vi "Rejestrator2_stare.vi"() -> ()   [LabVIEW 2014]
uses:
  C:/Users/user/Documents/Rudpol2/Kontrolki/GUI/AI_parametry.ctl
  C:/Users/user/Documents/Rudpol2/Kontrolki/GUI/AI_wartosc.ctl
  C:/Users/user/Documents/Rudpol2/Kontrolki/KartaDAQ/CONF AI HW config.ctl
  C:/Users/user/Documents/Rudpol2/Kontrolki/GUI/DI_aktywacja.ctl
  C:/Users/user/Documents/Rudpol2/Kontrolki/GUI/Encoder_parametry.ctl
  C:/Users/user/Documents/Rudpol2/Kontrolki/GUI/Encoder_chanel.ctl
  C:/Users/user/Documents/Rudpol2/Kontrolki/GUI/Enkoder Data.ctl
  C:/Users/user/Documents/Rudpol2/Kontrolki/GUI/Rejestracja_szybka.ctl
  C:/Users/user/Documents/Rudpol2/Kontrolki/GUI/Rejestracja_wolna.ctl
  C:/Users/user/Documents/Rudpol2/Kontrolki/GUI/RejWol_konfig.ctl
  C:/Users/user/Documents/Rudpol2/Kontrolki/GUI/RejWol_typ.ctl
  C:/Users/user/Documents/Rudpol2/Kontrolki/GUI/Wolna_WykrNum.ctl
  C:/Users/user/Documents/Rudpol2/Kontrolki/FVGs/FVG akcje podstawowa.ctl
  C:/Users/user/Documents/Rudpol2/Kontrolki/KartaDAQ/CONF digital channel config.ctl
  C:/Users/user/Documents/Rudpol2/Kontrolki/KartaDAQ/ACQ counter channel config.ctl
  C:/Users/user/Documents/Rudpol2/Kontrolki/KartaDAQ/ACQ all read tasks.ctl
  C:/Users/user/Documents/Rudpol2/Kontrolki/Przetwarzanie/Kanaly.ctl
  C:/Users/user/Documents/Rudpol2/Kontrolki/KartaDAQ/ACQ analog channel config new.ctl
  C:/Users/user/Documents/Rudpol2/Kontrolki/FVGs/TDMS FVG.ctl
  C:/Users/user/Documents/Rudpol2/Kontrolki/KartaDAQ/ACQ analog channel config.ctl
  C:/Users/user/Documents/Rudpol2/Kontrolki/FVGs/FVG akwizycje akcje.ctl
  C:/Users/user/Documents/Rudpol2/Kontrolki/FVGs/FVG GUI akcje.ctl
  C:/Users/user/Documents/Rudpol2/Kontrolki/FVGs/Referencje Mem akcje.ctl
  C:/Users/user/Documents/Rudpol2/Kontrolki/FVGs/TDMS Group dane FVG.ctl
  C:/Users/user/Documents/Rudpol2/Kontrolki/FVGs/TDMS File dane FVG.ctl
  C:/Users/user/Documents/Rudpol2/Kontrolki/FVGs/FVG Czas.ctl
  <vilib>/DAQmx/configure/task.llb/DAQmx Start Task.vi
  <vilib>/measure/NI_MABase.lvlib
panel:
  out "wolna delay":u32
  out "# elements in szybka queue":i32
  out "# elements in  wolna queue":i32
  out "Array":string[](array[string])
  out "Stan":string
  in  "Wykonujący":string="Marek" caption="Nazwa Pomiaru"
  in  "Obiekt":string="GUIDO" caption="Nazwa Pomiaru"
  out "Enk rozm":i32
  out "Boolean":bool
  out "Skala":dbl=100.0 format="%#_13g"
  out "acq czas":dbl=0.01953125
  out "Mnożniki wszystkie":dbl[](array[numeric])=[1.92, 1.92, 1.0, 1.0, 1.0, 1.0, 1.0, 1.0]
  out "Mnożniki out":dbl[](array[numeric])=[1.92, 1.92]
  in  "Tab Control":T1(tab)=enum."Konfiguracja"
  in  "Wykryj urządzenie":bool=TRUE
  out "AI HW conf real":T2[](array[typedef])
  in  "Urządzenie":tag="Dev1"
  in  "AI HW conf array in":T2[](array[typedef])
  out "Error Array":errorcluster[](array[cluster])
  out "Czasy Array":dbl[](array[numeric])
  in  "ZapiszAI_DI":bool
  in  "WczytajAI_DI":bool
  in  "Rejestracja wolna":T3={"WolnaStart"=FALSE, "WolnaPrzeglad"=FALSE, "Okres"=0.2, "Czas max"=3200.0, "WolnaKonfiguracja"=FALSE, "Rej.1"={"Typ rejestracji"=enum."Wprost", "Kanały"=[1], "Opis"="Rej.X", "Aktywny"=FALSE, "Wolna Wykr num"=0}, "Rej.2"={"Typ rejestracji"=enum."Wprost", "Kanały"=[1], "Opis"="Rej.X", "Aktywny"=FALSE, "Wolna Wykr num"=0}, "Rej.3"={"Typ rejestracji"=enum."Wprost", "Kanały"=[1], "Opis"="Rej.X", "Aktywny"=FALSE, "Wolna Wykr num"=0}, "Rej.4"={"Typ rejestracji"=enum."Wprost", "Kanały"=[1], "Opis"="Rej.X", "Aktywny"=FALSE, "Wolna Wykr num"=0}, "Rej.5"={"Typ rejestracji"=enum."Wprost", "Kanały"=[1], "Opis"="Rej.X", "Aktywny"=FALSE, "Wolna Wykr num"=0}, "Rej.6"={"Typ rejestracji"=enum."Wprost", "Kanały"=[1], "Opis"="Rej.X", "Aktywny"=FALSE, "Wolna Wykr num"=0}, "Rej.7"={"Typ rejestracji"=enum."Wprost", "Kanały"=[1], "Opis"="Rej.X", "Aktywny"=FALSE, "Wolna Wykr num"=0}, "Rej.8"={"Typ rejestracji"=enum."Wprost", "Kanały"=[1], "Opis"="Rej.X", "Aktywny"=FALSE, "Wolna Wykr num"=0}} {"Rej.8"."Wolna Wykr num" items=["Brak", "Wykres 1", "Wykres 2", "Wykres 3", "Wykres 4"]; "Rej.7"."Wolna Wykr num" items=["Brak", "Wykres 1", "Wykres 2", "Wykres 3", "Wykres 4"]; "Rej.6"."Wolna Wykr num" items=["Brak", "Wykres 1", "Wykres 2", "Wykres 3", "Wykres 4"]; "Rej.5"."Wolna Wykr num" items=["Brak", "Wykres 1", "Wykres 2", "Wykres 3", "Wykres 4"]; "Rej.4"."Wolna Wykr num" items=["Brak", "Wykres 1", "Wykres 2", "Wykres 3", "Wykres 4"]; "Rej.3"."Wolna Wykr num" items=["Brak", "Wykres 1", "Wykres 2", "Wykres 3", "Wykres 4"]; "Rej.2"."Wolna Wykr num" items=["Brak", "Wykres 1", "Wykres 2", "Wykres 3", "Wykres 4"]; "Rej.1"."Wolna Wykr num" items=["Brak", "Wykres 1", "Wykres 2", "Wykres 3", "Wykres 4"]}
  in  "Rejestracja szybka":T7={"SzybkaStart"=FALSE, "SzybkaPrzeglad"=FALSE, "Śledzenie"=enum."Migawka", "Czas"=4} {"Czas" scale=4.0..10.0}
  in  "Przemieszczenie":T8={"Wzorcowanie"=FALSE, "Zerowanie"=FALSE, "dT"=0.5, "Kanał"=enum."Kanał A", "Enkoder Data"={"d"=0.0, "v"=0.0, "a"=0.0}}
  in  "Kanały cyfrowe":T11={"DI1"=TRUE, "DI2"=FALSE, "DI3"=FALSE, "DI4"=FALSE, "DI1 Opis"="DI1", "DI2 Opis"="DI2", "DI3 Opis"="DI3", "DI4 Opis"="DI4", "DI1 Amplituda"=5.0, "DI2 Amplituda"=5.0, "DI3 Amplituda"=5.0, "DI4 Amplituda"=5.0}
  out "AI8":bool
  out "AI7":bool
  out "AI6":bool
  out "AI5":bool
  out "AI4":bool
  out "AI3":bool
  out "AI2":bool=TRUE
  out "AI1":bool=TRUE
  in  "Analog input":T12(tab)=enum."Kanał 8" caption="Wejścia Analogowe (konfiguracja)"
  in  "AI_parametry 1":T13={"Numer"=1, "Opis"="Kanał 1", "Zakres"=enum."3V", "Filtr"=FALSE, "Typ pomiaru"=enum."Wartość średnia", "Aktywny"=TRUE, "Wartość"={"X"="U", "[ ]"="V", "trans X"=1.0, "trans U"=1.0, "Z tabeli"=FALSE, "Opis"=""}} {"Numer" min=1 max=8 step=1}
  in  "AI_parametry 2":T13={"Numer"=1, "Opis"="Kanał 2", "Zakres"=enum."3V", "Filtr"=FALSE, "Typ pomiaru"=enum."Wartość średnia", "Aktywny"=TRUE, "Wartość"={"X"="U", "[ ]"="V", "trans X"=1.0, "trans U"=1.0, "Z tabeli"=FALSE, "Opis"=""}} {"Numer" min=1 max=8 step=1}
  in  "AI_parametry 3":T13={"Numer"=1, "Opis"="Kanał 3", "Zakres"=enum."1000V", "Filtr"=FALSE, "Typ pomiaru"=enum."Wartość średnia", "Aktywny"=FALSE, "Wartość"={"X"="U", "[ ]"="V", "trans X"=1.0, "trans U"=1.0, "Z tabeli"=FALSE, "Opis"=""}} {"Numer" min=1 max=8 step=1}
  in  "AI_parametry 4":T13={"Numer"=1, "Opis"="Kanał 4", "Zakres"=enum."1000V", "Filtr"=FALSE, "Typ pomiaru"=enum."Wartość średnia", "Aktywny"=FALSE, "Wartość"={"X"="U", "[ ]"="V", "trans X"=1.0, "trans U"=1.0, "Z tabeli"=FALSE, "Opis"=""}} {"Numer" min=1 max=8 step=1}
  in  "AI_parametry 5":T13={"Numer"=1, "Opis"="Kanał 5", "Zakres"=enum."1000V", "Filtr"=FALSE, "Typ pomiaru"=enum."Wartość średnia", "Aktywny"=FALSE, "Wartość"={"X"="U", "[ ]"="V", "trans X"=1.0, "trans U"=1.0, "Z tabeli"=FALSE, "Opis"=""}} {"Numer" min=1 max=8 step=1}
  in  "AI_parametry 6":T13={"Numer"=1, "Opis"="Kanał 6", "Zakres"=enum."1000V", "Filtr"=FALSE, "Typ pomiaru"=enum."Wartość średnia", "Aktywny"=FALSE, "Wartość"={"X"="U", "[ ]"="V", "trans X"=1.0, "trans U"=1.0, "Z tabeli"=FALSE, "Opis"=""}} {"Numer" min=1 max=8 step=1}
  in  "AI_parametry 7":T13={"Numer"=1, "Opis"="Kanał 7", "Zakres"=enum."1000V", "Filtr"=FALSE, "Typ pomiaru"=enum."Wartość średnia", "Aktywny"=FALSE, "Wartość"={"X"="U", "[ ]"="V", "trans X"=1.0, "trans U"=1.0, "Z tabeli"=FALSE, "Opis"=""}} {"Numer" min=1 max=8 step=1}
  in  "AI_parametry 8":T13={"Numer"=1, "Opis"="Kanał 8", "Zakres"=enum."1000V", "Filtr"=FALSE, "Typ pomiaru"=enum."Wartość średnia", "Aktywny"=FALSE, "Wartość"={"X"="U", "[ ]"="V", "trans X"=1.0, "trans U"=1.0, "Z tabeli"=FALSE, "Opis"=""}} {"Numer" min=1 max=8 step=1}
  in  "Edytuj Zapisane":bool
  in  "WolnyZapisz":bool
  in  "Nazwa Pomiaru W":string="Pomiar Wolny" caption="Nazwa Pomiaru"
  in  "Edytuj Wolny":bool
  out "Wolna data":waveform(dbl)[](graph)
  out "Wolna buf":waveform(dbl)[](graph)
  in  "Wolna STOP":bool
  in  "Zakres wysw wolna":dbl=30.0 caption="Zakres wyświetlania"
  out "Slide":dbl(slide) scale=0.0..4.0
  in  "Szybka ZAKONCZ":bool
  in  "Szybka STOP":bool
  out "Szybka":waveform(dbl)[](graph)=[{"t0"=timestamp(3529656835.064492 s since 1904-01-01), "dt"=0.0003125, "Y"=array[32000 elements], "attributes"=variant("Aktywny"=variant(bool TRUE), "NI_ChannelName"=variant(string "Kanał 1"), "NI_UnitDescription"=variant(string "Volts"), "NO"=variant(i32 0))}, {"t0"=timestamp(3529656835.064506 s since 1904-01-01), "dt"=0.0003125, "Y"=array[32000 elements], "attributes"=variant("Aktywny"=variant(bool TRUE), "NI_ChannelName"=variant(string "Kanał 1"), "NI_UnitDescription"=variant(string "Volts"), "NO"=variant(i32 1))}, {"t0"=timestamp(3529656835.0645204 s since 1904-01-01), "dt"=0.0003125, "Y"=array[32000 elements], "attributes"=variant("Aktywny"=variant(bool TRUE), "NI_ChannelName"=variant(string "Kanał 1"), "NI_UnitDescription"=variant(string "Volts"), "NO"=variant(i32 2))}, {"t0"=timestamp(3529656835.064534 s since 1904-01-01), "dt"=0.0003125, "Y"=array[32000 elements], "attributes"=variant("Aktywny"=variant(bool TRUE), "NI_ChannelName"=variant(string "Kanał 1"), "NI_UnitDescription"=variant(string "Volts"), "NO"=variant(i32 3))}, {"t0"=timestamp(3529656835.064548 s since 1904-01-01), "dt"=0.0003125, "Y"=array[32000 elements], "attributes"=variant("Aktywny"=variant(bool TRUE), "NI_ChannelName"=variant(string "Kanał 1"), "NI_UnitDescription"=variant(string "Volts"), "NO"=variant(i32 4))}, {"t0"=timestamp(3529656835.0645623 s since 1904-01-01), "dt"=0.0003125, "Y"=array[32000 elements], "attributes"=variant("Aktywny"=variant(bool TRUE), "NI_ChannelName"=variant(string "Kanał 1"), "NI_UnitDescription"=variant(string "Volts"), "NO"=variant(i32 5))}, {"t0"=timestamp(3529656835.064576 s since 1904-01-01), "dt"=0.0003125, "Y"=array[32000 elements], "attributes"=variant("Aktywny"=variant(bool TRUE), "NI_ChannelName"=variant(string "Kanał 1"), "NI_UnitDescription"=variant(string "Volts"), "NO"=variant(i32 6))}, {"t0"=timestamp(3529656835.0645905 s since 1904-01-01), "dt"=0.0003125, "Y"=array[32000 elements], "attributes"=variant("Aktywny"=variant(bool TRUE), "NI_ChannelName"=variant(string "Kanał 1"), "NI_UnitDescription"=variant(string "Volts"), "NO"=variant(i32 7))}, {"t0"=timestamp(3529656835.0646043 s since 1904-01-01), "dt"=0.0003125, "Y"=array[32000 elements], "attributes"=variant("Aktywny"=variant(bool TRUE), "NI_ChannelName"=variant(string "DI1"), "NI_UnitDescription"=variant(string "Volts"), "NO"=variant(i32 0))}, {"t0"=timestamp(3529656835.064618 s since 1904-01-01), "dt"=0.0003125, "Y"=array[32000 elements], "attributes"=variant("Aktywny"=variant(bool TRUE), "NI_ChannelName"=variant(string "DI2"), "NI_UnitDescription"=variant(string "Volts"), "NO"=variant(i32 1))}, {"t0"=timestamp(3529656835.0646324 s since 1904-01-01), "dt"=0.0003125, "Y"=array[32000 elements], "attributes"=variant("Aktywny"=variant(bool TRUE), "NI_ChannelName"=variant(string "DI3"), "NI_UnitDescription"=variant(string "Volts"), "NO"=variant(i32 2))}, {"t0"=timestamp(3529656835.0646462 s since 1904-01-01), "dt"=0.0003125, "Y"=array[32000 elements], "attributes"=variant("Aktywny"=variant(bool TRUE), "NI_ChannelName"=variant(string "D4"), "NI_UnitDescription"=variant(string "Volts"), "NO"=variant(i32 3))}, {"t0"=timestamp(0 s since 1904-01-01), "dt"=0.02, "Y"=[0.0, 0.0, 0.0, 0.0, 0.0, 0.0, 0.0, 0.0, 0.0, 0.0, 0.0, 0.0, 0.0, 0.0, 0.0, 0.0, 0.0, 0.0, 0.0, 0.0, 0.0, 0.0, 0.0, 0.0, 0.0, 0.0, 0.0, 0.0, 0.0, 0.0, 0.0, 0.0, 0.0, 0.0, 0.0, 0.0, 0.0, 0.0, 0.0, 0.0, 0.0, 0.0, 0.0, 0.0, 0.0, 0.0, 0.0, 0.0, 0.0, 0.0, 0.0, 0.0, 0.0, 0.0, 0.0, 0.0, 0.0, 0.0, 0.0, 0.0, 0.0, 0.0, 0.0, 0.0, 0.0, 0.0, 0.0, 0.0, 0.0, 0.0, 0.0, 0.0, 0.0, 0.0, 0.0, 0.0, 0.0, 0.0, 0.0, 0.0, 0.0, 0.0, 0.0, 0.0, 0.0, 0.0, 0.0, 0.0, 0.0, 0.0, 0.0, 0.0, 0.0, 0.0, 0.0, 0.0, 0.0, 0.0, 0.0, 0.0, 0.0, 0.0, 0.0, 0.0, 0.0, 0.0, 0.0, 0.0, 0.0, 0.0, 0.0, 0.0, 0.0, 0.0, 0.0, 0.0, 0.0, 0.0, 0.0, 0.0, 0.0, 0.0, 0.0, 0.0, 0.0, 0.0, 0.0, 0.0, 0.0, 0.0, 0.0, 0.0, 0.0, 0.0, 0.0, 0.0, 0.0, 0.0, 0.0, 0.0, 0.0, 0.0, 0.0, 0.0, 0.0, 0.0, 0.0, 0.0, 0.0, 0.0, 0.0, 0.0, 0.0, 0.0, 0.0, 0.0, 0.0, 0.0, 0.0, 0.0, 0.0, 0.0, 0.0, 0.0, 0.0, 0.0, 0.0, 0.0, 0.0, 0.0, 0.0, 0.0, 0.0, 0.0, 0.0, 0.0, 0.0, 0.0, 0.0, 0.0, 0.0, 0.0, 0.0, 0.0, 0.0, 0.0, 0.0, 0.0, 0.0, 0.0, 0.0, 0.0, 0.0, 0.0, 0.0, 0.0, 0.0, 0.0, 0.0, 0.0, 0.0, 0.0, 0.0, 0.0, 0.0, 0.0, 0.0, 0.0, 0.0, 0.0, 0.0, 0.0, 0.0, 0.0, 0.0, 0.0, 0.0, 0.0, 0.0, 0.0, 0.0, 0.0, 0.0, 0.0, 0.0, 0.0, 0.0, 0.0, 0.0, 0.0, 0.0, 0.0, 0.0, 0.0, 0.0, 0.0, 0.0, 0.0, 0.0, 0.0, 0.0, 0.0, 0.0, 0.0, 0.0, 0.0, 0.0, 0.0, 0.0, 0.0, 0.0, 0.0, 0.0, 0.0, 0.0, 0.0, 0.0, 0.0, 0.0, 0.0, 0.0, 0.0, 0.0, 0.0, 0.0, 0.0, 0.0, 0.0, 0.0, 0.0, 0.0, 0.0, 0.0, 0.0, 0.0, 0.0, 0.0, 0.0, 0.0, 0.0, 0.0, 0.0, 0.0, 0.0, 0.0, 0.0, 0.0, 0.0, 0.0, 0.0, 0.0, 0.0, 0.0, 0.0, 0.0, 0.0, 0.0, 0.0, 0.0, 0.0, 0.0, 0.0, 0.0, 0.0, 0.0, 0.0, 0.0, 0.0, 0.0, 0.0, 0.0, 0.0, 0.0, 0.0, 0.0, 0.0, 0.0, 0.0, 0.0, 0.0, 0.0, 0.0, 0.0, 0.0, 0.0, 0.0, 0.0, 0.0, 0.0, 0.0, 0.0, 0.0, 0.0, 0.0, 0.0, 0.0, 0.0, 0.0, 0.0, 0.0, 0.0, 0.0, 0.0, 0.0, 0.0, 0.0, 0.0, 0.0, 0.0, 0.0, 0.0, 0.0, 0.0, 0.0, 0.0, 0.0, 0.0, 0.0, 0.0, 0.0, 0.0, 0.0, 0.0, 0.0, 0.0, 0.0, 0.0, 0.0, 0.0, 0.0, 0.0, 0.0, 0.0, 0.0, 0.0, 0.0, 0.0, 0.0, 0.0, 0.0, 0.0, 0.0, 0.0, 0.0, 0.0, 0.0, 0.0, 0.0, 0.0, 0.0, 0.0, 0.0, 0.0, 0.0, 0.0, 0.0, 0.0, 0.0, 0.0, 0.0, 0.0, 0.0, 0.0, 0.0, 0.0, 0.0, 0.0, 0.0, 0.0, 0.0, 0.0, 0.0, 0.0, 0.0, 0.0, 0.0, 0.0, 0.0, 0.0, 0.0, 0.0, 0.0, 0.0, 0.0, 0.0, 0.0, 0.0, 0.0, 0.0, 0.0, 0.0, 0.0, 0.0, 0.0, 0.0, 0.0, 0.0, 0.0, 0.0, 0.0, 0.0, 0.0, 0.0, 0.0, 0.0, 0.0, 0.0, 0.0, 0.0, 0.0, 0.0, 0.0, 0.0, 0.0, 0.0, 0.0, 0.0, 0.0, 0.0, 0.0, 0.0, 0.0, 0.0, 0.0, 0.0, 0.0, 0.0, 0.0, 0.0, 0.0, 0.0, 0.0, 0.0, 0.0, 0.0, 0.0, 0.0, 0.0, 0.0, 0.0, 0.0, 0.0, 0.0, 0.0, 0.0, 0.0, 0.0, 0.0, 0.0, 0.0, 0.0, 0.0, 0.0, 0.0, 0.0, 0.0, 0.0, 0.0, 0.0, 0.0], "attributes"=variant("NI_ChannelName"=variant(string "Kanał A"))}]
  in  "Edytuj Szybki":bool
  in  "Zakres wysw szybka":dbl=5.0 caption="Zakres wyświetlania"
  in  "Nazwa Pomiaru S":string="Pomiar Szybki" caption="Nazwa Pomiaru"
  in  "SzybkiZapisz":bool
  out "DI4":bool
  out "DI3":bool
  out "DI2":bool
  out "DI1":bool caption="Stop"
  in  "Pokaż wszystkie":bool
  out "Kanał 8":dbl
  out "Kanał 7":dbl
  out "Kanał 6":dbl
  out "Kanał 5":dbl
  out "Kanał 4":dbl
  out "Kanał 3":dbl
  out "Kanał 2":dbl
  out "Kanał 1":dbl
  in  "StopBtn":bool
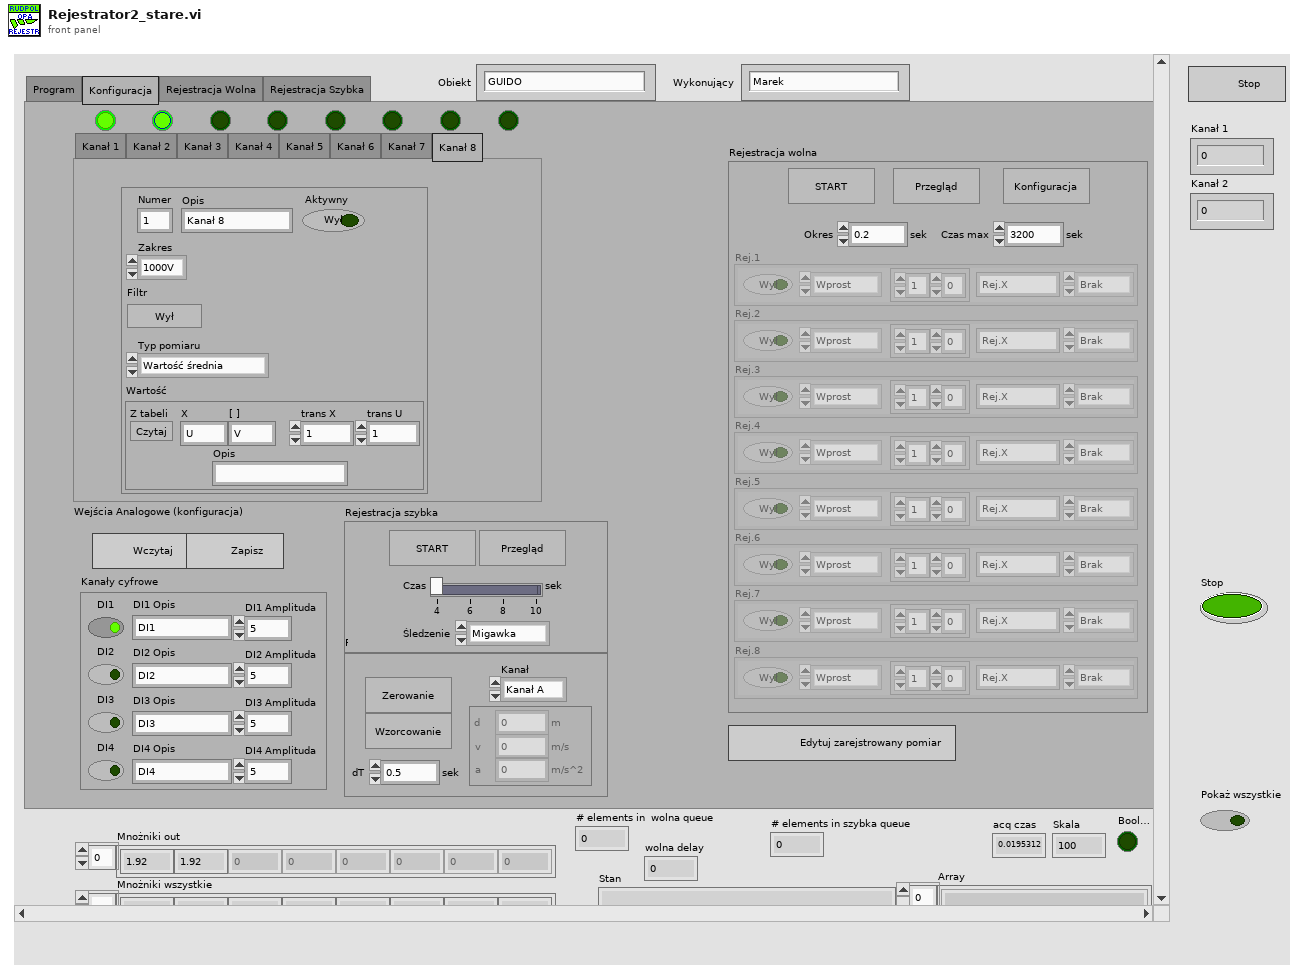
[diagram p1: front panel]
types:
  T1 = enum32{"Program", "Konfiguracja", "Rejestracja Wolna", "Rejestracja Szybka"}
  T2 = typedef "CONF AI HW config.ctl" = cluster{"res0":bool, "Div1":bool, "Div2":bool, "Mux1":bool, "Div3":bool, "Mux3":bool, "Mux2":bool, "res7":bool}
  T3 = typedef "Rejestracja_wolna.ctl" = cluster{"WolnaStart":bool, "WolnaPrzeglad":bool, "Okres":dbl, "Czas max":dbl, "WolnaKonfiguracja":bool, "Rej.1":T4, "Rej.2":T4, "Rej.3":T4, "Rej.4":T4, "Rej.5":T4, "Rej.6":T4, "Rej.7":T4, "Rej.8":T4}
  T4 = typedef "RejWol_konfig.ctl" = cluster{"Typ rejestracji":T5, "Kanały":i32[], "Opis":string, "Aktywny":bool, "Wolna Wykr num":T6}
  T5 = typedef "RejWol_typ.ctl" = enum16{"Wprost", "Moduł", "Kwadrat", "Iloczyn", "Faza"}
  T6 = typedef "Wolna_WykrNum.ctl" = u16
  T7 = typedef "Rejestracja_szybka.ctl" = cluster{"SzybkaStart":bool, "SzybkaPrzeglad":bool, "Śledzenie":enum16{"Obwiednia", "Migawka"}, "Czas":i32}
  T8 = typedef "Encoder_parametry.ctl" = cluster{"Wzorcowanie":bool, "Zerowanie":bool, "dT":dbl, "Kanał":T9, "Enkoder Data":T10}
  T9 = typedef "Encoder_chanel.ctl" = enum16{"Kanał A", "Kanał B"}
  T10 = typedef "Enkoder Data.ctl" = cluster{"d":dbl, "v":dbl, "a":dbl}
  T11 = typedef "DI_aktywacja.ctl" = cluster{"DI1":bool, "DI2":bool, "DI3":bool, "DI4":bool, "DI1 Opis":string, "DI2 Opis":string, "DI3 Opis":string, "DI4 Opis":string, "DI1 Amplituda":dbl, "DI2 Amplituda":dbl, "DI3 Amplituda":dbl, "DI4 Amplituda":dbl}
  T12 = enum32{"Kanał 1", "Kanał 2", "Kanał 3", "Kanał 4", "Kanał 5", "Kanał 6", "Kanał 7", "Kanał 8"}
  T13 = typedef "AI_parametry.ctl" = cluster{"Numer":u8, "Opis":string, "Zakres":enum16{"1000V", "300V", "30V", "3V", "0,3V"}, "Filtr":bool, "Typ pomiaru":enum16{"Wartość średnia", "Średnia wyprostowana", "Wartość skuteczna"}, "Aktywny":bool, "Wartość":T14}
  T14 = typedef "AI_wartosc.ctl" = cluster{"X":string, "[ ]":string, "trans X":dbl, "trans U":dbl, "Z tabeli":bool, "Opis":string}
  T15 = typedef "TDMS FVG.ctl" = enum16{"Konfig", "Dodaj Grupe", "Koniec"}
  T16 = typedef "ACQ analog channel config new.ctl" = cluster{"Analogs IN":string[], "Digitals IN":string[]}
  T17 = typedef "FVG akcje podstawowa.ctl" = enum16{"GET", "SET"}
  T18 = typedef "Kanaly.ctl" = cluster{"Analogowe":waveform(dbl)[], "Cyfrowe":waveform(dbl)[], "Zwarcie":waveform(dbl)[], "Enkoder":waveform(dbl)[]}
  T19 = typedef "ACQ all read tasks.ctl" = cluster{"Enkoder X ref":refnum<k21>, "Enkoder Y ref":refnum<k21>, "Generator ref":refnum<k21>, "Analog ref":refnum<k21>}
  T20 = typedef "ACQ analog channel config.ctl" = cluster{"Analog IN":string, "Digital IN":string, "Cont IN":string}
  T21 = typedef "ACQ counter channel config.ctl" = cluster{"Enkoder X":string, "Enkoder Y":string, "Generator":string, "Generator OUT":string}
  T22 = typedef "CONF digital channel config.ctl" = cluster{"SEnable":string, "SData":string, "SClock":string}
  T23 = typedef "FVG akwizycje akcje.ctl" = enum16{"GET", "GETr", "SET"}
  T24 = typedef "Referencje Mem akcje.ctl" = enum16{"GET", "SET"}
  T25 = typedef "FVG GUI akcje.ctl" = enum16{"GET", "SET AI Aktywny", "SET DI Aktywny"}
  T26 = typedef "DAQ card Dane.ctl" = cluster{"ID":string, "Typ":string, "Serial":u32}
  T27 = typedef "CONF Digital Refnum.ctl" = cluster{"Sen Ref out":refnum<k21>, "Data Ref out":refnum<k21>}
  T28 = enum16{"Sine Wave", "Triangle Wave", "Square Wave", "Sawtooth Wave"}
  T29 = typedef "TDMS Group dane FVG.ctl" = cluster{"Nazwa":string, "L.Kanalow":string}
  T30 = typedef "TDMS File dane FVG.ctl" = cluster{"Katalog":path, "Kopalnia":string, "Wykonujący":string}
  T31 = typedef "eventsource.ctl" = u32
  T32 = typedef "FVG Czas.ctl" = u16
  T33 = enum16{"Wartość średnia", "Średnia wyprostowana", "Wartość skuteczna"}
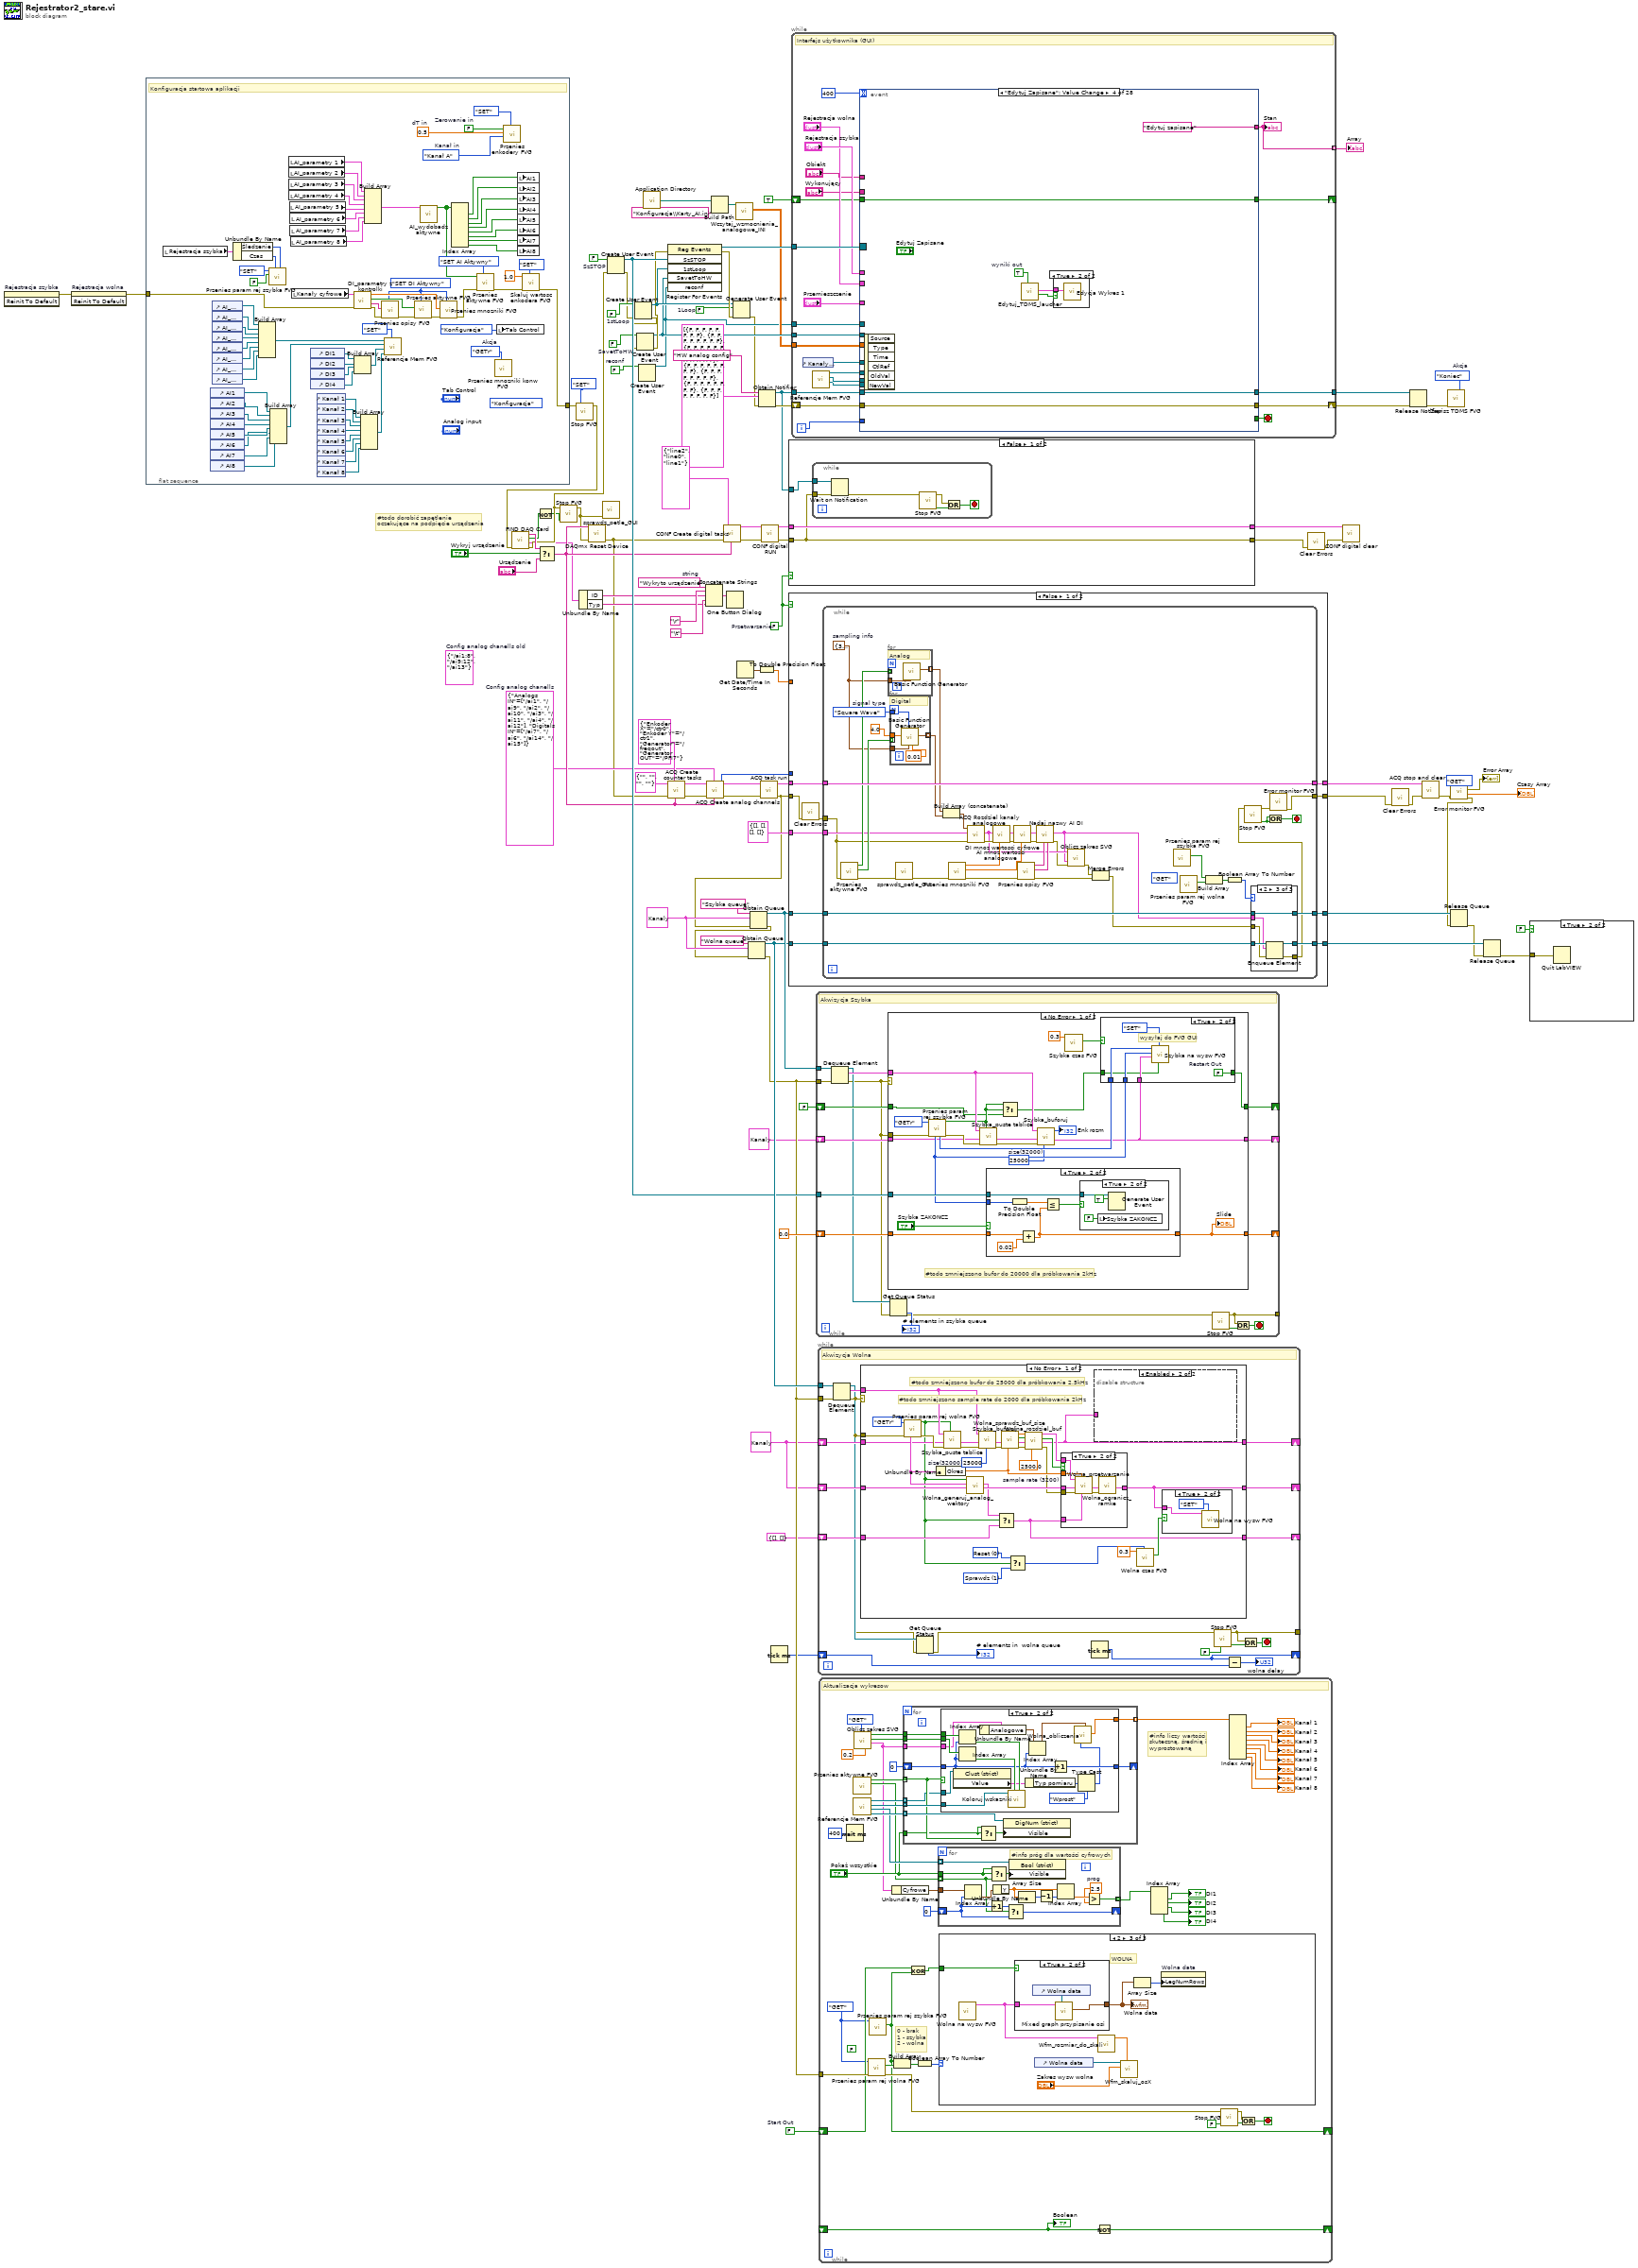
[diagram p0: block diagram]
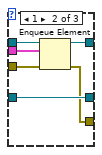
[diagram p4: hidden frame]
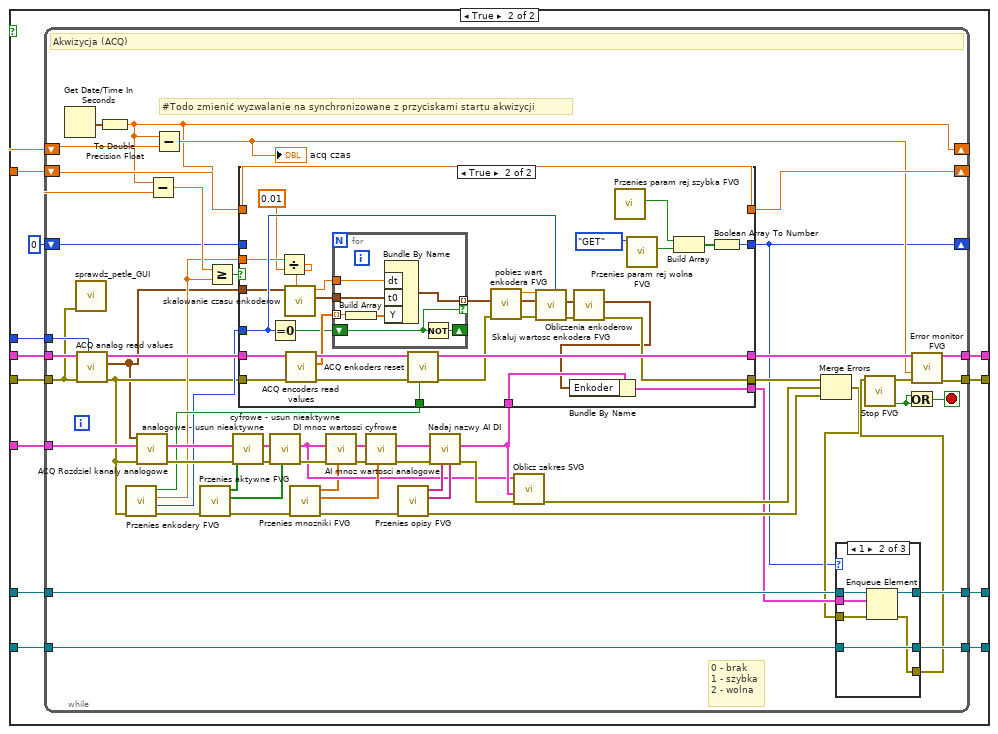
[diagram p5: hidden frame]
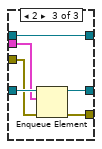
[diagram p7: hidden frame]
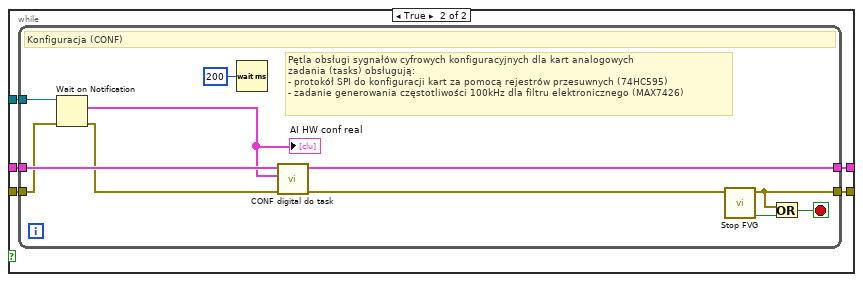
[diagram p9: hidden frame]
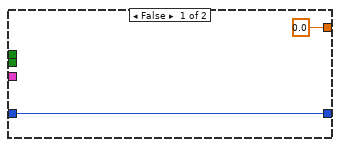
[diagram p10: hidden frame]
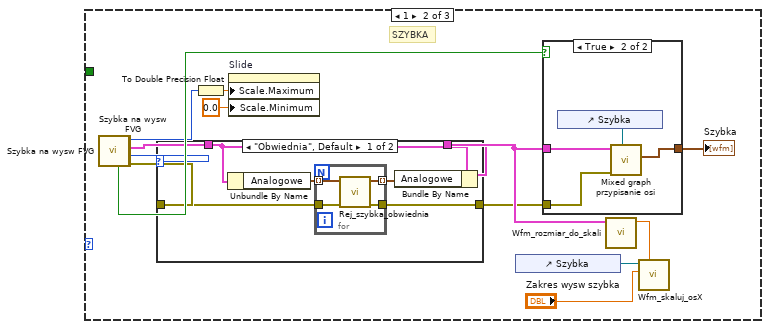
[diagram p12: hidden frame]
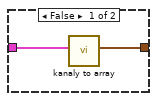
[diagram p13: hidden frame]
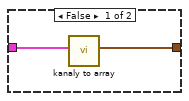
[diagram p15: hidden frame]
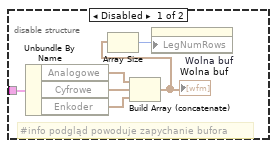
[diagram p16: hidden frame]
diagram:
  w3 = FALSE  # Przetwarzanie
  w13 = TDMS_FVG."Koniec"  # Akcja
  w17 = FALSE  # reconf
  w22 = T16 {"Analogs IN"=["/ai1", "/ai9", "/ai2", "/ai10", "/ai3", "/ai11", "/ai4", "/ai12"], "Digitals IN"=["/ai7", "/ai6", "/ai14", "/ai15"]}  # Config analog chanells
  w29 = "Wykryto urządzenie"  # string
  w41 = FALSE  # Start Out
  w50 = T18 data[32432B] ("Data out")
  w57 = FALSE  # SavetToHW
  w58 = FALSE  # 1Loop
  w61 = FALSE  # 1stLoop
  w63 = FALSE  # SzSTOP
  w71 = T18 data[32432B] ("Kanaly")
  (unwired) T20 {"Analog IN"="/ai1:8", "Digital IN"="/ai9:12", "Cont IN"="/ai13"}  # Config analog chanells old
  # "#todo dorobić zapętlenie\noczekujące na podpięcie urządzenia"
  n1 = invoke on="Rejestracja szybka" class="Clust (strict)" method="Reinit To Default"() -> (error out=w24:errorcluster)  [unwired: 3 in, 2 out]
  n2 = invoke on="Rejestracja wolna" class="Clust (strict)" method="Reinit To Default"(error in=w24) -> (error out=w23:errorcluster)  [unwired: 2 in, 2 out]
  n3 = flat-sequence {
    tunnel: [w155] -> w84
    tunnel: w23 -> [w106]
    frame #0 {
      w100 = FVG_akwizycje_akcje."GETr"  # Akcja
      w119 = Encoder_chanel."Kanał A"  # Kanał in
      w118 = 0.5  # dT in
      w117 = FALSE  # Zerowanie in
      (unwired) T1."Konfiguracja" ("Tab Control")
      w108 = FVG_GUI_akcje."SET DI Aktywny" ("Akcja (Get)")
      # "Konfiguracja startowa aplikacji"
      n4 = local read "Rejestracja szybka"() -> (w132:T7)
      n5 = control-ref of="AI1"() -> (w141:refnum<vi>)
      n6 = control-ref of="AI2"() -> (w140:refnum<vi>)
      n7 = control-ref of="AI3"() -> (w139:refnum<vi>)
      n8 = control-ref of="AI4"() -> (w138:refnum<vi>)
      n9 = control-ref of="AI5"() -> (w137:refnum<vi>)
      n10 = control-ref of="AI6"() -> (w136:refnum<vi>)
      n11 = control-ref of="AI7"() -> (w135:refnum<vi>)
      n12 = control-ref of="AI8"() -> (w134:refnum<vi>)
      n13 = control-ref of="AI_parametry 1"() -> (w150:refnum<vi>)
      n14 = control-ref of="AI_parametry 2"() -> (w149:refnum<vi>)
      n15 = control-ref of="AI_parametry 3"() -> (w148:refnum<vi>)
      n16 = control-ref of="AI_parametry 4"() -> (w147:refnum<vi>)
      n17 = control-ref of="AI_parametry 5"() -> (w146:refnum<vi>)
      n18 = control-ref of="AI_parametry 6"() -> (w145:refnum<vi>)
      n19 = control-ref of="AI_parametry 7"() -> (w144:refnum<vi>)
      n20 = control-ref of="AI_parametry 8"() -> (w143:refnum<vi>)
      n21 = Unbundle By Name(w132) -> ("Śledzenie"=w131:enum16{"Obwiednia", "Migawka"}, "Czas"=w130:i32)
      n22 = Build Array(w150, w149, w148, w147, w146, w145, w144, w143) -> (w151:refnum<vi>[])
      n23 = call "Przenies param rej szybka FVG.vi"("Śledzenie In"=w131, "Czas In"=w130, "Start In"=FALSE, "Akcja"=FVG_akwizycje_akcje."SET") -> ()  [unwired: 3 in, 5 out]
      n24 = Build Array(w141, w140, w139, w138, w137, w136, w135, w134) -> (w142:refnum<vi>[])
      n25 = local read "AI_parametry 1"() -> (w175:T13)
      n26 = local read "AI_parametry 2"() -> (w174:T13)
      n27 = local read "AI_parametry 3"() -> (w173:T13)
      n28 = local read "AI_parametry 4"() -> (w172:T13)
      n29 = local read "AI_parametry 5"() -> (w171:T13)
      n30 = local read "AI_parametry 6"() -> (w170:T13)
      n31 = local read "AI_parametry 7"() -> (w169:T13)
      n32 = local read "AI_parametry 8"() -> (w168:T13)
      n33 = local read "Kanały cyfrowe"() -> (w107:T11)
      n34 = control-ref of="DI1"() -> (w104:refnum<vi>)
      n35 = control-ref of="DI2"() -> (w103:refnum<vi>)
      n36 = control-ref of="DI3"() -> (w102:refnum<vi>)
      n37 = control-ref of="DI4"() -> (w101:refnum<vi>)
      n38 = control-ref of="Kanał 1"() -> (w128:refnum<vi>)
      n39 = control-ref of="Kanał 2"() -> (w127:refnum<vi>)
      n40 = control-ref of="Kanał 3"() -> (w126:refnum<vi>)
      n41 = control-ref of="Kanał 4"() -> (w125:refnum<vi>)
      n42 = control-ref of="Kanał 5"() -> (w124:refnum<vi>)
      n43 = control-ref of="Kanał 6"() -> (w123:refnum<vi>)
      n44 = control-ref of="Kanał 7"() -> (w122:refnum<vi>)
      n45 = control-ref of="Kanał 8"() -> (w121:refnum<vi>)
      n46 = call "DI_parametry z kontrolki.vi"("error in (no error)"=w106, "Kanały cyfrowe in"=w107) -> ("error out"=w112:errorcluster, "Opisy out"=w111:string[], "Aktywne out"=w110:bool[], "Mnożniki out"=w109:dbl[])  [unwired: 6 in]
      n47 = Build Array(w104, w103, w102, w101) -> (w105:refnum<vi>[])
      n48 = Build Array(w128, w127, w126, w125, w124, w123, w122, w121) -> (w120:refnum<vi>[])
      n49 = Build Array(w175, w174, w173, w172, w171, w170, w169, w168) -> (w158:T13[])
      n50 = call "Przenies opisy FVG.vi"("Akcja (Get)"=w108, "error in (no error)"=w112, "DI opisy in"=w111) -> ("error out"=w114:errorcluster)  [unwired: 6 in, 2 out]
      n51 = call "Referencje Mem FVG.vi"("Akcja"=Referencje_Mem_akcje."SET" ("Akcja (GET)"), "AI wskazniki array in"=w120, "DI wartosci array in"=w105, "AI aktywne array in"=w142, "AI_param array in"=w151) -> ()  [unwired: 3 in, 4 out]
      n52 = call "Przenies aktywne FVG.vi"("Akcja (Get)"=w108, "error in (no error)"=w114, "DI Aktywne in"=w110) -> ("error out"=w115:errorcluster)  [unwired: 6 in, 2 out]
      n53 = call "AI_wydobadz aktywne.vi"("AI param array in"=w158) -> ("Aktywne Array out"=w157:bool[])  [unwired: 8 in, 2 out]
      n54 = call "Przenies mnozniki FVG.vi"("Akcja (Get)"=w108, "error in (no error)"=w115, "DI Mnozniki in"=w109) -> ("error out"=w113:errorcluster)  [unwired: 6 in, 2 out]
      n55 = Index Array(array=w157) -> (element #1=w167:bool, element #2=w166:bool, element #3=w165:bool, element #4=w164:bool, element #5=w163:bool, element #6=w162:bool, element #7=w161:bool, element #8=w160:bool)  [unwired: 8 in]
      n56 = call "Przenies aktywne FVG.vi"("Akcja (Get)"=FVG_GUI_akcje."SET AI Aktywny", "error in (no error)"=w113, "AI Aktywne in"=w157) -> ("error out"=w156:errorcluster)  [unwired: 6 in, 2 out]
      n57 = call "Przenies mnozniki konw FVG.vi"("Akcja (GET)"=w100) -> ()  [unwired: 9 in, 2 out]
      n58 = local write "Tab Control"(T1."Konfiguracja" ("Tab Control")) -> ()
      n59 = call "Przenies enkodery FVG.vi"("Akcja (Get)"=FVG_akcje_podstawowa."SET", "Kanał in"=w119, "dT in"=w118, "Zerowanie in"=w117) -> ()  [unwired: 4 in, 4 out]
      n60 = local write "AI1"(w167) -> ()
      n61 = local write "AI2"(w166) -> ()
      n62 = local write "AI3"(w165) -> ()
      n63 = local write "AI4"(w164) -> ()
      n64 = local write "AI5"(w163) -> ()
      n65 = local write "AI6"(w162) -> ()
      n66 = local write "AI7"(w161) -> ()
      n67 = local write "AI8"(w160) -> ()
      n68 = call "Skaluj wartosc enkodera FVG.vi"("Akcja (GET)"=FVG_akcje_podstawowa."SET", "error in (no error)"=w156, "Skala"=1.0) -> ("error out"=w155:errorcluster)  [unwired: 7 in, 1 out]
    }
  }
  n69 = call "Stop FVG.vi"("Akcja (GET)"=FVG_akcje_podstawowa."SET", "error in (no error)"=w84) -> ("error out"=w35:errorcluster)  [unwired: 8 in, 1 out]
  n70 = call "FIND DAQ Card.vi"("Error In"=w35) -> ("Error Out"=w34:errorcluster, "Karta"=w30:T26, "Znaleziono?"=w32:bool, "DAQmx Device Name"=w38:tag)  [unwired: 6 in, 1 out]
  n71 = Not(x=w32) -> (.not. x?=w33:bool)
  n72 = Select(t=w38, s="Wykryj urządzenie", f="Urządzenie") -> (s? t:f=w36:tag)
  n73 = call "Stop FVG.vi"("Stop in (F)"=w33, "error in (no error)"=w34) -> ("error out"=w6:errorcluster)  [unwired: 8 in, 1 out]
  n74 = Unbundle By Name(w30) -> ("ID"=w27:string, "Typ"=w25:string)
  n75 = call <vilib>:"DAQmx Reset Device.vi"("device in"=w36, "error in"=w6) -> ("error out"=w7:errorcluster)  [unwired: 13 in]
  n76 = call "sprawdz_petle_GUI.vi"("error in (no error)"=w6) -> ()  [unwired: 9 in, 2 out]
  n77 = Create User Event(user event datatype=w63, error in=w34) -> (user event=w62:refnum<user-event>, error out=w60:errorcluster)
  n78 = Create User Event(user event datatype=w61, error in=w60) -> (user event=w54:refnum<user-event>, error out=w55:errorcluster)
  n79 = Create User Event(user event datatype=w57, error in=w55) -> (user event=w53:refnum<user-event>, error out=w56:errorcluster)
  n80 = Create User Event(user event datatype=w17) -> (user event=w16:refnum<user-event>)  [unwired: 1 in, 1 out]
  n81 = call <vilib>:"Application Directory.vi"() -> ("Application Directory"=w20:path)
  n82 = register-events(error in=w56, w62, w54, w53, w16) -> (reference out=w64:refnum<event-registration>, error out=w59:errorcluster)  [unwired: 1 in]
  n83 = call "ACQ Create counter tasks.vi"("device in"=w36, "Config Counter channels"=T21 {"Enkoder X"="/ctr0", "Enkoder Y"="/ctr1", "Generator"="/freqout", "Generator OUT"="/PFI7"}, "error in (no error)"=w7, "All Read tasks in"=T19 {"Enkoder X ref"="", "Enkoder Y ref"="", "Generator ref"="", "Analog ref"=""}) -> ("error out"=w8:errorcluster, "All Read tasks out"=w85:T19)  [unwired: 5 in, 1 out]
  n84 = Concatenate Strings(w29, "\r", w27, "\t", w25) -> (w31:string)
  n85 = call "ACQ Create analog channels.vi"("device in"=w36, "Config analog chanells new"=w22, "error in (no error)"=w8, "All Read tasks in"=w85) -> ("error out"=w10:errorcluster, "All Read tasks out"=w83:T19, "samples per channel"=w81:i32)  [unwired: 4 in, 1 out]
  n86 = Build Path(base path=w20, name or relative path="Konfiguracja\\Karty_AI.ini") -> (appended path=w19:path)
  n87 = call "CONF Create digital tasks.vi"("device in"=w36, "Config Digital Channels"=T22 {"SEnable"="line2", "SData"="line0", "SClock"="line1"}, "error in (no error)"=w7) -> ("error out"=w5:errorcluster, "Digital ref out"=w97:T27)  [unwired: 7 in]
  n88 = One Button Dialog(message=w31) -> ()  [unwired: 1 in, 1 out]
  n89 = Generate User Event(user event=w54, event data cluster=w58, error in=w59) -> (error out=w11:errorcluster)  [unwired: 1 in, 1 out]
  n90 = call "Wczytaj_wzmocnienia_analogowe_INI.vi"("Path ini"=w19) -> ("Wzmocnienia"=w18:dbl[][])  [unwired: 9 in, 1 out]
  n91 = Get Date/Time In Seconds() -> (seconds since 1Jan1904=w75:timestamp)
  n92 = To Double Precision Float(number=w75) -> (double precision float=w74:dbl)
  n93 = Obtain Notifier(name (unnamed)="HW analog config", notification data type=T2[] [{"res0"=FALSE, "Div1"=FALSE, "Div2"=FALSE, "Mux1"=FALSE, "Div3"=FALSE, "Mux3"=FALSE, "Mux2"=FALSE, "res7"=FALSE}, {"res0"=FALSE, "Div1"=FALSE, "Div2"=FALSE, "Mux1"=FALSE, "Div3"=FALSE, "Mux3"=FALSE, "Mux2"=FALSE, "res7"=FALSE}, {"res0"=FALSE, "Div1"=FALSE, "Div2"=FALSE, "Mux1"=FALSE, "Div3"=FALSE, "Mux3"=FALSE, "Mux2"=FALSE, "res7"=FALSE}, {"res0"=FALSE, "Div1"=FALSE, "Div2"=FALSE, "Mux1"=FALSE, "Div3"=FALSE, "Mux3"=FALSE, "Mux2"=FALSE, "res7"=FALSE}, {"res0"=FALSE, "Div1"=FALSE, "Div2"=FALSE, "Mux1"=FALSE, "Div3"=FALSE, "Mux3"=FALSE, "Mux2"=FALSE, "res7"=FALSE}, {"res0"=FALSE, "Div1"=FALSE, "Div2"=FALSE, "Mux1"=FALSE, "Div3"=FALSE, "Mux3"=FALSE, "Mux2"=FALSE, "res7"=FALSE}, {"res0"=FALSE, "Div1"=FALSE, "Div2"=FALSE, "Mux1"=FALSE, "Div3"=FALSE, "Mux3"=FALSE, "Mux2"=FALSE, "res7"=FALSE}, {"res0"=FALSE, "Div1"=FALSE, "Div2"=FALSE, "Mux1"=FALSE, "Div3"=FALSE, "Mux3"=FALSE, "Mux2"=FALSE, "res7"=FALSE}] ("AI HW conf array in"), error in (no error)=w11) -> (notifier out=w89:refnum<notifier>, error out=w94:errorcluster)  [unwired: 1 in, 1 out]
  n94 = call "ACQ task run.vi"("error in (no error)"=w10, "All Read tasks in"=w83) -> ("error out"=w9:errorcluster, "All Read tasks out"=w82:T19)  [unwired: 7 in, 1 out]
  n95 = Obtain Queue(name (unnamed)="Szybka queue", element data type=w71, error in (no error)=w9) -> (queue out=w67:refnum<queue>, error out=w51:errorcluster)  [unwired: 2 in, 1 out]
  n96 = Obtain Queue(name (unnamed)="Wolna queue", element data type=w71, error in (no error)=w51) -> (queue out=w66:refnum<queue>, error out=w52:errorcluster)  [unwired: 2 in, 1 out]
  n97 = call "CONF digital RUN.vi"("error in (no error)"=w5, "Digital ref in"=w97) -> ("error out"=w98:errorcluster, "Digital ref out"=w96:T27)  [unwired: 8 in]
  n98 = Tick Count (ms)() -> (millisecond timer value=w4:u32)
  n99 = case shown="False" w3 {
    tunnel: w82 -> [w181 w262]
    tunnel: w81 -> [_ w261]
    tunnel: [w182 w260] -> w80
    tunnel: [w180 w259] -> w79
    tunnel: w74 -> [_ w258]
    tunnel: [w184 w257] -> w70
    tunnel: [w186 w256] -> w69
    tunnel: w67 -> [w183 w255]
    tunnel: w66 -> [w185 w254]
    tunnel: T18 {"Analogowe"=[], "Cyfrowe"=[], "Zwarcie"=[], "Enkoder"=[]} ("Kanaly") -> [w179 w253]
    tunnel: w9 -> [w178 w251]
    frame False {
      n100 = call <vilib>:"Clear Errors.vi"("error in (no error)"=w178) -> ("error out"=w177:errorcluster)  [unwired: 5 in, 1 out]
      n101 = while {
        tunnel: [w228] -> w186
        tunnel: w185 -> [w227]
        tunnel: [w226] -> w184
        tunnel: w183 -> [w225]
        tunnel: [w224] -> w182
        tunnel: w181 -> [w224]
        tunnel: [w195] -> w180
        tunnel: w177 -> [w198]
        tunnel: w179 -> [w210]
        stop <- w193 stop-if-true
        w191 = T28."Square Wave"  # signal type
        w192 = cluster{"Fs":dbl, "#s":dbl} {"Fs"=3200.0, "#s"=32.0}  # sampling info
        (unwired) FVG_akwizycje_akcje."GET" ("Akcja")
        n102 = call "Przenies aktywne FVG.vi"("error in (no error)"=w198) -> ("error out"=w188:errorcluster, "DI Aktywne out"=w217:bool[], "AI Aktywne out"=w218:bool[])  [unwired: 8 in]
        n103 = for {
          tunnel: w218 -> [_] mode=indexing
          tunnel: [w235] -> w216 mode=indexing
          tunnel: w192 -> [w234]
          # "Analog"
          n104 = call <vilib>:"Basic Function Generator.vi"("sampling info"=w234) -> ("signal out"=w235:waveform(dbl))  [unwired: 8 in, 2 out]
        }
        n105 = for {
          tunnel: w217 -> [_] mode=indexing
          tunnel: [w233] -> w215 mode=indexing
          tunnel: w192 -> [w232]
          tunnel: w191 -> [w231]
          tunnel: 4.0 -> [w229]
          # "Digital"
          n106 = call <vilib>:"Basic Function Generator.vi"("square wave duty cycle (%)"=0.01, "sampling info"=w232, "signal type"=w231, "amplitude"=w229) -> ("signal out"=w233:waveform(dbl))  [unwired: 5 in, 2 out]
        }
        n107 = call "sprawdz_petle_GUI.vi"("error in (no error)"=w188) -> ("error out"=w189:errorcluster)  [unwired: 9 in, 1 out]
        n108 = Build Array (concatenate)(w216, w215) -> (w211:waveform(dbl)[])
        n109 = call "Przenies mnozniki FVG.vi"("error in (no error)"=w189) -> ("error out"=w219:errorcluster, "DI Mnozniki out"=w209:dbl[], "AI Mnozniki out"=w212:dbl[])  [unwired: 8 in]
        n110 = call "ACQ Rozdziel kanaly analogowe.vi"("error in (no error)"=w198, "Kanaly in"=w210, "data"=w211) -> ("error out"=w207:errorcluster, "Kanaly out"=w204:T18)  [unwired: 7 in]
        n111 = call "AI mnoz wartosci analogowe.vi"("Mnozniki in"=w212, "error in (no error)"=w207, "Kanaly in"=w204) -> ("error out"=w208:errorcluster, "Kanaly out"=w213:T18)  [unwired: 6 in, 1 out]
        n112 = call "DI mnoz wartosci cyfrowe.vi"("Mnozniki in"=w209, "error in (no error)"=w208, "Kanaly in"=w213) -> ("error out"=w202:errorcluster, "Kanaly out"=w214:T18)  [unwired: 6 in, 1 out]
        n113 = call "Przenies opisy FVG.vi"("error in (no error)"=w219) -> ("error out"=w200:errorcluster, "DI opisy out"=w205:string[], "AI opisy out"=w206:string[])  [unwired: 8 in]
        n114 = call "Nadaj nazwy AI DI.vi"("DI opisy in"=w205, "AI opisy in"=w206, "error in (no error)"=w202, "Kanaly in"=w214) -> ("error out"=w203:errorcluster, "Kanaly out"=w187:T18)  [unwired: 6 in]
        n115 = call "Oblicz zakres SVG.vi"("error in (no error)"=w203, "Przetw in"=w187, "Kanaly nieprzetw in"=w204) -> ("error out"=w201:errorcluster)  [unwired: 5 in, 3 out]
        n116 = Merge Errors(w201, w200) -> (w199:errorcluster)
        n117 = call "Przenies param rej szybka FVG.vi"() -> ("Start Out"=w221:bool)  [unwired: 7 in, 4 out]
        n118 = call "Przenies param rej wolna FVG.vi"() -> ("Start Out"=w223:bool)  [unwired: 8 in, 3 out]
        n119 = Build Array(w221, w223) -> (w222:bool[])
        n120 = Boolean Array To Number(Boolean array=w222) -> (number=w220:u32)
        n121 = case shown="2" w220 {
          tunnel: w225 -> [w238 w244 w246]
          tunnel: w227 -> [w237 w241 w250]
          tunnel: [w238 w243 w246] -> w226
          tunnel: [w237 w241 w249] -> w228
          tunnel: w199 -> [w236 w242 w247]
          tunnel: [w236 w240 w248] -> w194
          tunnel: w187 -> [_ w239 w245]
          frame 0, Default {
          }
          frame 1 {
            n122 = Enqueue Element(queue=w244, element=w239, error in (no error)=w242) -> (queue out=w243:refnum<queue>, error out=w240:errorcluster)  [unwired: 1 in, 1 out]
          }
          frame 2 {
            n123 = Enqueue Element(queue=w250, element=w245, error in (no error)=w247) -> (queue out=w249:refnum<queue>, error out=w248:errorcluster)  [unwired: 1 in, 1 out]
          }
        }
        n124 = call "Stop FVG.vi"("error in (no error)"=w194) -> ("Stop out"=w197:bool, "error out"=w196:errorcluster)  [unwired: 9 in]
        n125 = Or(x=w197, y=w197) -> (x .or. y?=w193:bool)
        n126 = call "Error monitor FVG.vi"("error in (no error)"=w196) -> ("error out"=w195:errorcluster)  [unwired: 8 in, 2 out]
      }
    }
    frame True {
      n127 = while {
        tunnel: w251 -> [w264]
        tunnel: w262 -> [w316]
        tunnel: w261 -> [w318]
        tunnel: [w275] -> w259
        tunnel: [w314] -> w260
        shift-right: [w309] -> _
        shift-left: w258 -> [w308]
        shift-right: [w269] -> _
        shift-left: w258 -> [w307]
        tunnel: w255 -> [w285]
        tunnel: w254 -> [w284]
        tunnel: [w294] -> w257
        tunnel: [w293] -> w256
        tunnel: w253 -> [w282]
        shift-right: [w268] -> _
        shift-left: u32 0 -> [w267]
        stop <- w317 stop-if-true
        # "#Todo zmienić wyzwalanie na synchronizowane z przyciskami startu akwizycji"
        # "0 - brak\n1 - szybka\n2 - wolna"
        # "Akwizycja (ACQ)"
        n128 = Get Date/Time In Seconds() -> (seconds since 1Jan1904=w312:timestamp)
        n129 = call "sprawdz_petle_GUI.vi"("error in (no error)"=w264) -> ()  [unwired: 9 in, 2 out]
        n130 = call "ACQ analog read values.vi"("samples per channel"=w318, "error in (no error)"=w264, "Tasks ref in"=w316) -> ("error out"=w265:errorcluster, "data"=w263:waveform(dbl)[], "Tasks ref out"=w315:T19)  [unwired: 6 in]
        n131 = To Double Precision Float(number=w312) -> (double precision float=w269:dbl)
        n132 = call "Przenies enkodery FVG.vi"("error in (no error)"=w265) -> ("error out"=w297:errorcluster, "Kanał out"=w295:T9, "dT out"=w278:dbl, "Zerowanie out"=w296:bool)  [unwired: 7 in]
        n133 = call "ACQ Rozdziel kanaly analogowe.vi"("error in (no error)"=w265, "Kanaly in"=w282, "data"=w263) -> ("error out"=w303:errorcluster, "Kanaly out"=w306:T18)  [unwired: 7 in]
        n134 = Subtract(x=w269, y=w308) -> (x-y=w311:dbl)
        n135 = Subtract(x=w269, y=w307) -> (x-y=w274:dbl)
        "acq czas" <- w274
        n136 = call "Przenies aktywne FVG.vi"("error in (no error)"=w297) -> ("error out"=w301:errorcluster, "DI Aktywne out"=w304:bool[], "AI Aktywne out"=w305:bool[])  [unwired: 8 in]
        n137 = Greater Or Equal?(x=w311, y=w278) -> (x >= y?=w310:bool)
        n138 = call "analogowe - usun nieaktywne.vi"("Kanaly aktywne"=w305, "error in (no error)"=w303, "Kanaly in"=w306) -> ("error out"=w302:errorcluster, "Kanaly out"=w273:T18)  [unwired: 7 in]
        n139 = call "cyfrowe - usun nieaktywne.vi"("Kanaly aktywne"=w304, "error in (no error)"=w302, "Kanaly in"=w273) -> ("error out"=w300:errorcluster, "Kanaly out"=w272:T18)  [unwired: 7 in]
        n140 = call "Przenies mnozniki FVG.vi"("error in (no error)"=w301) -> ("error out"=w291:errorcluster, "DI Mnozniki out"=w298:dbl[], "AI Mnozniki out"=w266:dbl[])  [unwired: 8 in]
        n141 = call "AI mnoz wartosci analogowe.vi"("Mnozniki in"=w266, "error in (no error)"=w300, "Kanaly in"=w272) -> ("error out"=w299:errorcluster, "Kanaly out"=w279:T18)  [unwired: 6 in, 1 out]
        n142 = call "DI mnoz wartosci cyfrowe.vi"("Mnozniki in"=w298, "error in (no error)"=w299, "Kanaly in"=w279) -> ("error out"=w289:errorcluster, "Kanaly out"=w288:T18)  [unwired: 6 in, 1 out]
        n143 = call "Przenies opisy FVG.vi"("error in (no error)"=w291) -> ("error out"=w290:errorcluster, "DI opisy out"=w286:string[], "AI opisy out"=w287:string[])  [unwired: 8 in]
        n144 = call "Nadaj nazwy AI DI.vi"("DI opisy in"=w286, "AI opisy in"=w287, "error in (no error)"=w289, "Kanaly in"=w288) -> ("error out"=w281:errorcluster, "Kanaly out"=w277:T18)  [unwired: 6 in]
        n145 = case shown="True" w310 {
          tunnel: w265 -> [w337 w370]
          tunnel: w315 -> [w338 w369]
          tunnel: [w337 w353] -> w283
          tunnel: [w338 w367] -> w314
          tunnel: w308 -> [w336 _]
          tunnel: [w336 w368] -> w309
          tunnel: w269 -> [_ w368]
          tunnel: w296 -> [_ w364]
          tunnel: w295 -> [_ w356]
          tunnel: w278 -> [_ w341]
          tunnel: w277 -> [w335 w352]
          tunnel: [w335 w350] -> w271
          tunnel: [w334 w346] -> w268
          tunnel: w267 -> [w334 _]
          tunnel: w263 -> [_ w344]
          frame False {
          }
          frame True {
            n146 = Equal To 0?(x=w356) -> (x = 0?=w362:bool)
            n147 = Divide(x=w341, y=0.01) -> (x/y=w340:dbl)
            n148 = call "skalowanie czasu enkoderow.vi"("mnoznik"=w340, "data"=w344) -> ("t0"=w342:timestamp, "dT out"=w343:dbl)  [unwired: 8 in]
            n149 = call "ACQ encoders read values.vi"("error in (no error)"=w370, "Tasks ref in"=w369) -> ("error out"=w366:errorcluster, "Encoders out"=w363:dbl[], "Tasks ref out"=w365:T19)  [unwired: 7 in]
            n150 = for {
              tunnel: w363 -> [w377] mode=indexing
              tunnel: [w375] -> w360 mode=indexing if=w373
              shift-right: [w374] -> _
              shift-left: w362 -> [w373]
              tunnel: w343 -> [w372]
              tunnel: w342 -> [w371]
              n151 = Build Array(w377) -> (w376:dbl[])
              n152 = Bundle By Name("dt"=w372, "t0"=w371, "Y"=w376) -> (w375:waveform(dbl))  [unwired: 1 in]
              n153 = Not(x=w373) -> (.not. x?=w374:bool)
            }
            n154 = call "ACQ enkoders reset.vi"("Reset"=w364, "error in (no error)"=w366, "Tasks ref in"=w365) -> ("error out"=w359:errorcluster, "Tasks ref out"=w367:T19)  [unwired: 7 in]
            n155 = call "pobiez wart enkodera FVG.vi"("error in (no error)"=w359, "Impulsy In"=w360) -> ("error out"=w361:errorcluster, "Impulsy Out wfm"=w358:waveform(dbl)[], "Impulsy Out"=w357:dbl)  [unwired: 6 in, 1 out]
            n156 = call "Skaluj wartosc enkodera FVG.vi"("Kanał in"=w356, "error in (no error)"=w361, "Impulsy In"=w358, "Skala"=w357) -> ("error out"=w354:errorcluster, "Impulsy Out"=w355:waveform(dbl)[])  [unwired: 6 in]
            n157 = call "Obliczenia enkoderow.vi"("error in (no error)"=w354, "Enkoder in"=w355) -> ("error out"=w353:errorcluster, "Enkoder out"=w351:waveform(dbl)[])  [unwired: 8 in]
            n158 = Bundle By Name(cluster=w352, "Enkoder"=w351) -> (w350:T18)
            n159 = call "Przenies param rej szybka FVG.vi"() -> ("Start Out"=w345:bool)  [unwired: 7 in, 4 out]
            n160 = call "Przenies param rej wolna FVG.vi"("Akcja"=FVG_akwizycje_akcje."GET") -> ("Start Out"=w349:bool)  [unwired: 7 in, 3 out]
            n161 = Build Array(w345, w349) -> (w347:bool[])
            n162 = Boolean Array To Number(Boolean array=w347) -> (number=w346:u32)
          }
        }
        n163 = call "Oblicz zakres SVG.vi"("error in (no error)"=w281, "Przetw in"=w277, "Kanaly nieprzetw in"=w272) -> ("error out"=w280:errorcluster)  [unwired: 5 in, 3 out]
        n164 = Merge Errors(w283, w280, w290) -> (w270:errorcluster)
        n165 = case shown="1" w268 {
          tunnel: w285 -> [w321 w327 w328]
          tunnel: w284 -> [w320 w323 w333]
          tunnel: w271 -> [_ w326 w329]
          tunnel: [w321 w325 w328] -> w294
          tunnel: [w320 w323 w332] -> w293
          tunnel: w270 -> [w319 w324 w330]
          tunnel: [w319 w322 w331] -> w292
          frame 0, Default {
          }
          frame 1 {
            n166 = Enqueue Element(queue=w327, element=w326, error in (no error)=w324) -> (queue out=w325:refnum<queue>, error out=w322:errorcluster)  [unwired: 1 in, 1 out]
          }
          frame 2 {
            n167 = Enqueue Element(queue=w333, element=w329, error in (no error)=w330) -> (queue out=w332:refnum<queue>, error out=w331:errorcluster)  [unwired: 1 in, 1 out]
          }
        }
        n168 = call "Stop FVG.vi"("error in (no error)"=w292) -> ("Stop out"=w313:bool, "error out"=w276:errorcluster)  [unwired: 9 in]
        n169 = Or(x=w313, y=w313) -> (x .or. y?=w317:bool)
        n170 = call "Error monitor FVG.vi"("error in (no error)"=w276, "acq czas"=w274) -> ("error out"=w275:errorcluster)  [unwired: 7 in, 2 out]
      }
    }
  }
  n171 = case shown="False" w3 {
    tunnel: w98 -> [w378 w391]
    tunnel: w96 -> [w380 w390]
    tunnel: [w380 w389] -> w95
    tunnel: w89 -> [w379 w388]
    tunnel: [w378 w387] -> w88
    frame False {
      n172 = while {
        tunnel: w379 -> [w386]
        tunnel: w378 -> [w382]
        stop <- w381 stop-if-true
        n173 = Wait on Notification(notifier=w386, error in (no error)=w382) -> (error out=w383:errorcluster)  [unwired: 2 in, 3 out]
        n174 = call "Stop FVG.vi"("error in (no error)"=w383) -> ("Stop out"=w385:bool, "error out"=w384:errorcluster)  [unwired: 9 in]
        n175 = Or(x=w384, y=w385) -> (x .or. y?=w381:bool)
      }
    }
    frame True {
      n176 = while {
        tunnel: w391 -> [w397]
        tunnel: w390 -> [w401]
        tunnel: [w394] -> w387
        tunnel: [w400] -> w389
        tunnel: w388 -> [w398]
        stop <- w393 stop-if-true
        # "Pętla obsługi sygnałów cyfrowych konfiguracyjnych dla kart analogowych\nzadania (tasks) obsługują:\n- protokół SPI do konfiguracji kart za pomocą rejestrów przesuwnych (74HC595)\n- zadanie generowania częstotliwości 100kHz dla filtru elektronicznego (MAX7426)"
        # "Konfiguracja (CONF)"
        n177 = Wait on Notification(notifier=w398, error in (no error)=w397) -> (notification=w392:T2[], error out=w396:errorcluster)  [unwired: 2 in, 2 out]
        "AI HW conf real" <- w392
        n178 = Wait (ms)(milliseconds to wait=u32 200) -> ()  [unwired: 1 out]
        n179 = call "CONF digital do task.vi"("error in (no error)"=w396, "AI HW conf array in"=w392, "Digital ref in"=w401) -> ("error out"=w399:errorcluster, "Digital ref out"=w400:T27)  [unwired: 6 in, 1 out]
        n180 = call "Stop FVG.vi"("error in (no error)"=w399) -> ("Stop out"=w395:bool, "error out"=w394:errorcluster)  [unwired: 9 in]
        n181 = Or(x=w394, y=w395) -> (x .or. y?=w393:bool)
      }
    }
  }
  n182 = while {
    shift-right: [w424] -> w91
    shift-left: w94 -> [w423]
    tunnel: w89 -> [w422]
    tunnel: [w421] -> w90
    tunnel: w64 -> [w420]
    tunnel: w53 -> [w413]
    tunnel: w18 -> [w411]
    tunnel: w16 -> [w409]
    shift-right: [w407] -> _
    shift-left: TRUE -> [w408]
    tunnel: [w404] -> w12 mode=indexing
    i -> [w403]
    stop <- w425 stop-if-true
    # "Interfejs użytkownika (GUI)"
    n183 = control-ref of="Kanały cyfrowe"() -> (w414:refnum<vi>)
    n184 = call "Referencje Mem FVG.vi"() -> ("DI wartosci array out"=w410:refnum<vi>[], "AI aktywne array out"=w415:refnum<vi>[], "AI_param array out"=w416:refnum<vi>[])  [unwired: 8 in, 1 out]
    n185 = event shown="[3] \"Edytuj Zapisane\": Value Change" {
      selector: w420 -> [_ _ _ _ _ _ _ _ _ _ _ _ _ _ _ _ _ _ _ _ _ _ _ _ _ _ _ _]
      dyn-events: _ -> [_ _ _ _ _ _ _ _ _ _ _ _ _ _ _ _ _ _ _ _ _ _ _ _ _ _ _ _]
      timeout: 400 -> [_ _ _ _ _ _ _ _ _ _ _ _ _ _ _ _ _ _ _ _ _ _ _ _ _ _ _ _]
      tunnel: [_ _ _ _ _ w544 _ _ _ _ _ _ _ _ _ _ _ _ _ _ _ _ _ _ _ _ _ _] -> w425
      tunnel: [w438 w455 w506 w530 w537 w546 w556 w565 w579 w627 w647 w663 w686 w707 w728 w749 w770 w791 w812 w829 w846 w859 w879 w894 w903 w913 w925 w935] -> w424
      tunnel: w423 -> [w438 w455 w506 w530 w537 w545 w556 w565 w606 w628 w648 w653 w687 w708 w729 w750 w771 w792 w813 w828 w847 w859 w879 w894 w904 w914 w926 w938]
      tunnel: w422 -> [w437 w454 w505 w529 w536 w542 w555 w564 w608 w634 w649 w668 w693 w714 w735 w756 w777 w798 w819 w840 w844 w858 w878 w893 w908 w917 w930 w949]
      tunnel: [w437 w454 w505 w529 w536 w542 w555 w564 w607 w634 w649 w668 w693 w714 w735 w756 w777 w798 w819 w840 w843 w858 w878 w893 w908 w917 w930 w949] -> w421
      tunnel: "Rejestracja szybka" -> [_ _ _ _ _ _ _ _ w570 _ _ _ _ _ _ _ _ _ _ _ _ w853 _ _ w906 _ _ _]
      tunnel: "Rejestracja wolna" -> [_ w453 _ _ w535 _ w552 w561 w571 _ _ _ _ _ _ _ _ _ _ _ _ _ w866 _ _ w915 _ _]
      tunnel: w416 -> [_ _ _ _ _ _ _ _ _ _ _ _ w691 w712 w733 w754 w775 w796 w817 w826 _ _ _ _ _ _ w924 w941]
      tunnel: w415 -> [_ _ _ _ _ _ _ _ _ _ _ _ _ _ _ _ _ _ _ _ _ _ _ _ _ _ _ w940]
      tunnel: w414 -> [_ _ _ _ _ _ _ _ _ _ _ _ _ _ _ _ _ _ _ _ _ _ _ _ _ _ w923 w942]
      tunnel: w413 -> [_ _ _ _ _ _ _ _ _ _ _ _ _ _ _ _ _ _ _ _ _ _ _ _ _ _ _ w936]
      tunnel: "Przemieszczenie" -> [w436 _ _ _ _ _ _ _ _ w624 _ _ _ _ _ _ _ _ _ _ _ _ _ _ _ _ _ _]
      tunnel: w411 -> [_ _ _ _ _ _ _ _ w568 _ _ _ _ _ _ _ _ _ _ _ _ _ _ _ _ _ _ _]
      tunnel: w410 -> [_ _ _ _ _ _ _ _ _ _ _ w655 _ _ _ _ _ _ _ _ _ _ _ _ _ _ _ _]
      tunnel: w409 -> [_ _ _ _ _ _ _ _ _ _ _ _ w680 w701 w722 w743 w764 w785 w806 w827 _ _ _ _ _ _ _ _]
      tunnel: w408 -> [w431 w452 w504 w528 w533 w541 w549 w558 w567 w621 w641 w651 w677 w698 w719 w740 w761 w782 w803 w824 w842 w849 w862 w889 w901 w910 w922 w932]
      tunnel: [w431 w451 w503 w528 w533 w541 w549 w558 w567 w621 w641 w651 w677 w698 w719 w740 w761 w782 w803 w824 w842 w849 w862 w889 w901 w910 w922 w932] -> w407
      tunnel: "Wykonujący" -> [_ w450 w492 _ _ _ _ _ _ _ _ _ _ _ _ _ _ _ _ _ _ _ _ _ _ _ _ _]
      tunnel: "Obiekt" -> [_ w449 w493 _ _ _ _ _ _ _ _ _ _ _ _ _ _ _ _ _ _ _ _ _ _ _ _ _]
      tunnel: ["Timeout" "Edytuj Wolny" "Edytuj Szybki" "Edytuj zapisane" "Rej Wolna.Wolna Konfig" "StopBtn" "Rej wolna Okres" "Wolna.Czas max" "Konfig Analog" "przemieszczenie wzorcowanie" "przemieszczenie" "cyfrowe konfig" "AI przetwornik" "AI przetwornik" "AI przetwornik" "AI przetwornik" "AI przetwornik" "AI przetwornik" "AI przetwornik" "AI przetwornik" "AI HW konfig" "Szybka Start" "Wolna Start" "Tab ctrl" "Szybka stop, SzSTOP" "Wolna Stop" "ZapiszAI_DI" "WczytajAI_DI"] -> w404
      tunnel: w403 -> [w427 _ _ _ _ _ _ _ _ _ _ _ _ _ _ _ _ _ _ _ _ _ _ _ _ _ _ _]
      event Timeout {
        n186 = event-data() -> ()  [unwired: 1 in, 3 out]
        n187 = Less?(x=4, y=w427) -> (x < y?=w428:bool)
        n188 = case shown="True" w428 {
          tunnel: [w439 w440] -> w429
          frame False {
            w439 = TRUE  # Stan
          }
          frame True {
            w441 = FVG_akcje_podstawowa."GET"  # Akcja (SET)
            n189 = call "sprawdz_petle_GUI.vi"("Akcja (SET)"=w441) -> ("Stan"=w440:bool)  [unwired: 9 in, 1 out]
          }
        }
        n190 = call "Enk Data przenies FVG.vi"("Akcja (SET)"=FVG_akcje_podstawowa."GET", "Enkoder Data in"=T10 {"d"=0.0, "v"=0.0, "a"=0.0}) -> ("Enkoder Data out"=w434:T10)  [unwired: 8 in, 1 out]
        n191 = Bundle By Name(cluster=w436, "Enkoder Data"=w434) -> (w435:T8)
        n192 = case shown="False" w429 {
          frame False {
            w442 = "Błąd"  # button name ("OK")
            w443 = "Akwizycja zatrzymana\nzrestartuj program!"  # message
            n193 = One Button Dialog(message=w443, button name ("OK")=w442) -> ()  [unwired: 1 out]
          }
          frame True {
          }
        }
        n194 = local write "Przemieszczenie"(w435) -> ()
      }
      event "Edytuj Wolny", "WolnyZapisz": Value Change {
        # "#todo czemu wywala"
        n195 = event-data() -> ("OldVal"=w447:bool, "NewVal"=w446:bool)  [unwired: 1 in, 4 out]
        n196 = Not Equal?(x=w447, y=w446) -> (x != y?=w445:bool)
        n197 = case shown="True" w445 {
          tunnel: w453 -> [_ w471]
          tunnel: w452 -> [w456 w462]
          tunnel: [w456 w461] -> w451
          tunnel: w450 -> [_ w459]
          tunnel: w449 -> [_ w458]
          tunnel: "Edytuj Wolny" -> [_ w457]
          frame False {
          }
          frame True {
            w465 = T29 {"Nazwa"="", "L.Kanalow"=""}  # Group Data
            w466 = TDMS_FVG."Dodaj Grupe"  # Akcja
            n198 = case shown="True" w462 {
              selector: w462 -> [w476 _]
              tunnel: [w476 FALSE] -> w461
              tunnel: [w475 w487] -> w460
              tunnel: w459 -> [_ w478]
              tunnel: w458 -> [_ w477]
              frame False {
                w475 = errorcluster {"status"=FALSE, "code"=0, "source"=""}  # no error
              }
              frame True {
                w481 = T30 {"Katalog"=path "", "Kopalnia"="", "Wykonujący"=""}  # File Data
                w484 = TRUE  # Uwzględnij czas (F)
                # "#info pierwsze użycie, konfiguracja"
                n199 = call <vilib>:"Application Directory.vi"() -> ("Application Directory"=w485:path)
                n200 = call "generuj_nazwe_pliku.vi"("Uwzględnij czas (F)"=w484, "Nazwa bazowa"="TDMS\\TDMS_", "Application Directory"=w485) -> ("error out"=w483:errorcluster, "appended path"=w479:path)  [unwired: 7 in]
                n201 = Bundle By Name(cluster=w481, "Kopalnia"=w477, "Wykonujący"=w478, "Katalog"=w479) -> (w480:T30)
                n202 = call "Zapisz TDMS FVG.vi"("Aktywacja"=TRUE, "Akcja"=TDMS_FVG."Konfig", "error in (no error)"=w483, "File Data"=w480) -> ("error out"=w487:errorcluster)  [unwired: 6 in, 1 out]
              }
            }
            n203 = Bundle By Name(cluster=w471, "WolnaPrzeglad"=FALSE ("SzybkaPrzeglad")) -> ()  [unwired: 1 out]
            n204 = Bundle By Name(cluster=w465, "Nazwa"="Nazwa Pomiaru W") -> (w464:T29)
            n205 = call "Wolna na wysw FVG.vi"("error in (no error)"=w460) -> ("error out"=w470:errorcluster, "Wolna out"=w469:T18)  [unwired: 9 in]
            n206 = call "Zapisz TDMS FVG.vi"("Akcja"=w466, "error in (no error)"=w470, "Group Data"=w464, "Przebiegi in"=w469) -> ("error out"=w467:errorcluster, "Przebiegi out"=w468:T18)  [unwired: 6 in]
            n207 = case shown="True" w457 {
              tunnel: w468 -> [_ w474]
              tunnel: w467 -> [_ w473]
              frame False {
              }
              frame True {
                n208 = call "Edycja Wykres 1.vi"("error in (no error)"=w473, "Data in"=w474) -> ()  [unwired: 9 in, 1 out]
              }
            }
          }
        }
      }
      event "Edytuj Szybki", "SzybkiZapisz": Value Change {
        w496 = T29 {"Nazwa"="", "L.Kanalow"=""}  # Group Data
        w497 = TDMS_FVG."Dodaj Grupe"  # Akcja
        n209 = event-data() -> ()  [unwired: 1 in, 6 out]
        n210 = case shown="True" w504 {
          selector: w504 -> [w510 _]
          tunnel: [w510 FALSE] -> w503
          tunnel: [w509 w521] -> w498
          tunnel: w493 -> [_ w512]
          tunnel: w492 -> [_ w511]
          frame False {
            w509 = errorcluster {"status"=FALSE, "code"=0, "source"=""}  # no error
          }
          frame True {
            w515 = T30 {"Katalog"=path "", "Kopalnia"="", "Wykonujący"=""}  # File Data
            w518 = TRUE  # Uwzględnij czas (F)
            # "#info pierwsze użycie, konfiguracja"
            n211 = call <vilib>:"Application Directory.vi"() -> ("Application Directory"=w519:path)
            n212 = call "generuj_nazwe_pliku.vi"("Uwzględnij czas (F)"=w518, "Nazwa bazowa"="TDMS\\TDMS_", "Application Directory"=w519) -> ("error out"=w517:errorcluster, "appended path"=w513:path)  [unwired: 7 in]
            n213 = Bundle By Name(cluster=w515, "Kopalnia"=w512, "Wykonujący"=w511, "Katalog"=w513) -> (w514:T30)
            n214 = call "Zapisz TDMS FVG.vi"("Aktywacja"=TRUE, "Akcja"=TDMS_FVG."Konfig", "error in (no error)"=w517, "File Data"=w514) -> ("error out"=w521:errorcluster)  [unwired: 6 in, 1 out]
          }
        }
        n215 = Bundle By Name(cluster=w496, "Nazwa"="Nazwa Pomiaru S") -> (w494:T29)
        n216 = call "Szybka na wysw FVG.vi"("error in (no error)"=w498) -> ("error out"=w500:errorcluster, "Bufor out"=w501:T18)  [unwired: 6 in, 3 out]
        n217 = call "Zapisz TDMS FVG.vi"("Akcja"=w497, "error in (no error)"=w500, "Group Data"=w494, "Przebiegi in"=w501) -> ("error out"=w499:errorcluster, "Przebiegi out"=w502:T18)  [unwired: 6 in]
        n218 = case shown="True" "Edytuj Szybki" {
          tunnel: w502 -> [_ w508]
          tunnel: w499 -> [_ w507]
          frame False {
          }
          frame True {
            n219 = call "Edycja Wykres 1.vi"("error in (no error)"=w507, "Data in"=w508) -> ()  [unwired: 9 in, 1 out]
          }
        }
      }
      event "Edytuj Zapisane": Value Change {
        w526 = TRUE  # wyniki out
        n220 = event-data() -> ()  [unwired: 1 in, 6 out]
        n221 = call "Edytuj_TDMS_laucher.vi"("wyniki out"=w526) -> ("OK?"=w524:bool, "Przebiegi"=w525:T18)  [unwired: 9 in]
        n222 = case shown="True" w524 {
          tunnel: w525 -> [_ w531]
          frame False {
          }
          frame True {
            n223 = call "Edycja Wykres 1.vi"("Data in"=w531) -> ()  [unwired: 10 in, 1 out]
          }
        }
      }
      event Value Change {
        n224 = event-data() -> ("NewVal"=w534:bool)  [unwired: 1 in, 5 out]
        n225 = case shown="True" w534 {
          tunnel: w535 -> [_ w539]
          frame False {
          }
          frame True {
            n226 = call "Rejestracja_konfiguracja.vi"("WolnaIn"=w539) -> ("WolnaOut"=w538:T3)  [unwired: 9 in, 1 out]
            n227 = local write "Rejestracja wolna"(w538) -> ()
          }
        }
      }
      event "StopBtn": Value Change {
        n228 = event-data() -> ()  [unwired: 1 in, 6 out]
        n229 = call "Stop FVG.vi"("Akcja (GET)"=FVG_akcje_podstawowa."SET", "Stop in (F)"="StopBtn", "error in (no error)"=w545) -> ("Stop out"=w544:bool, "error out"=w546:errorcluster)  [unwired: 7 in]
      }
      event Value Change {
        n230 = event-data() -> ("NewVal"=w551:dbl)  [unwired: 1 in, 5 out]
        n231 = Multiply(x=w551, y=16000.0) -> (x*y=w554:dbl)
        n232 = Bundle By Name(cluster=w552, "Czas max"=w554, "Okres"=w551) -> (w550:T3)
        n233 = local write "Rejestracja wolna"(w550) -> ()
      }
      event Value Change {
        n234 = event-data() -> ("NewVal"=w560:dbl)  [unwired: 1 in, 5 out]
        n235 = Divide(x=w560, y=16000.0) -> (x/y=w563:dbl)
        n236 = Bundle By Name(cluster=w561, "Okres"=w563, "Czas max"=w560) -> (w559:T3)
        n237 = local write "Rejestracja wolna"(w559) -> ()
      }
      event Value Change; User Event {
        w581 = FVG_GUI_akcje."SET AI Aktywny" ("Akcja")
        # "#todo dodać reakcję na wszystkie elementy konfiguracji kanałów"
        # "zmienia konfigurację kart analogowych w przystawce\npo włączeniu filtru lub zmianie zakresu\nna wybranym kanale analogowym"
        n238 = event-data() -> ("Source"=w569:T31)  [unwired: 1 in]
        n239 = case shown="25" w569 {
          tunnel: w571 -> [_ w610]
          tunnel: w570 -> [_ w609]
          frame 0, Default {
          }
          frame 25 {
            w613 = 1.0  # Skala
            w612 = FVG_akwizycje_akcje."SET" ("Akcja")
            n240 = Unbundle By Name(w610) -> ("WolnaStart"=w615:bool)
            n241 = Unbundle By Name(w609) -> ("Śledzenie"=w616:enum16{"Obwiednia", "Migawka"}, "Czas"=w617:i32, "SzybkaStart"=w619:bool)
            n242 = call "Przenies param rej wolna FVG.vi"("Wolna In"=w610, "Start In"=w615, "Akcja"=w612) -> ("error out"=w618:errorcluster)  [unwired: 5 in, 3 out]
            n243 = call "Przenies param rej szybka FVG.vi"("Śledzenie In"=w616, "Czas In"=w617, "error in (no error)"=w618, "Start In"=w619, "Akcja"=w612) -> ("error out"=w614:errorcluster)  [unwired: 2 in, 4 out]
            n244 = call "Skaluj wartosc enkodera FVG.vi"("Akcja (GET)"=FVG_akcje_podstawowa."SET", "error in (no error)"=w614, "Skala"=w613) -> ()  [unwired: 7 in, 2 out]
          }
        }
        n245 = Build Array("AI_parametry 1", "AI_parametry 2", "AI_parametry 3", "AI_parametry 4", "AI_parametry 5", "AI_parametry 6", "AI_parametry 7", "AI_parametry 8") -> (w587:T13[])
        n246 = call "AI_wydobadz aktywne.vi"("AI param array in"=w587) -> ("error out"=w585:errorcluster, "AI param aktywne out"=w582:T13[], "Aktywne Array out"=w586:bool[])  [unwired: 8 in]
        n247 = call "AI generuj wektor konfiguracji kart.vi"("AI_param in"=w587) -> ("HW konfig"=w605:T2[])  [unwired: 9 in, 1 out]
        n248 = Send Notification(notification=w605, notifier=w608, error in (no error)=w606) -> (notifier out=w607:refnum<notifier>, error out=w596:errorcluster)
        n249 = call "AI_Oblicz mnozniki teoret.vi"("Mnozniki"=w568, "error in (no error)"=w585, "AI param aktywne in"=w582, "Aktywne Array in"=w586) -> ("error out"=w577:errorcluster, "Mnożniki out"=w576:dbl[], "AI param aktywne out"=w575:T13[], "Aktywne Array out"=w574:bool[], "Mnożniki wszystkie out"=→"Mnożniki wszystkie":dbl[])  [unwired: 3 in]
        n250 = call "AI_wydobadz opisy.vi"("AI param aktywne in"=w582) -> ("AI opisy out"=w578:string[])  [unwired: 9 in, 1 out]
        n251 = call "AI mnoz wartosci z przetw.vi"("error in (no error)"=w577, "Mnożniki in"=w576, "AI param aktywne in"=w575, "Aktywne Array in"=w574) -> ("Mnożniki out"=w572:dbl[], "Aktywne Array out"=w573:bool[])  [unwired: 3 in, 3 out]
        "Mnożniki out" <- w572
        n252 = call "Przenies aktywne FVG.vi"("Akcja (Get)"=w581, "error in (no error)"=w596, "AI Aktywne in"=w573) -> ("error out"=w583:errorcluster)  [unwired: 6 in, 2 out]
        n253 = call "Przenies mnozniki FVG.vi"("Akcja (Get)"=w581, "error in (no error)"=w583, "AI Mnozniki in"=w572) -> ("error out"=w580:errorcluster)  [unwired: 6 in, 2 out]
        n254 = Index Array(array=w573) -> (element #1=→"AI1":bool, element #2=→"AI2":bool, element #3=→"AI3":bool, element #4=→"AI4":bool, element #5=→"AI5":bool, element #6=→"AI6":bool, element #7=→"AI7":bool, element #8=→"AI8":bool)  [unwired: 8 in]
        n255 = call "Przenies opisy FVG.vi"("Akcja (Get)"=w581, "error in (no error)"=w580, "AI opisy in"=w578) -> ("error out"=w579:errorcluster)  [unwired: 6 in, 2 out]
      }
      event Value Change {
        w622 = FALSE  # Wzorcowanie
        n256 = event-data() -> ()  [unwired: 1 in, 6 out]
        n257 = call "pobiez wart enkodera FVG.vi"("Akcja (Pobrano)"=enum16{"Pobierz", "Pobrano", "Czekaj"}."Pobierz", "error in (no error)"=w628) -> ("error out"=w632:errorcluster)  [unwired: 6 in, 3 out]
        n258 = while {
          tunnel: w632 -> [w637]
          tunnel: [w636] -> w631
          tunnel: [w635] -> w626
          stop <- w638 stop-if-true
          n259 = call "pobiez wart enkodera FVG.vi"("Akcja (Pobrano)"=enum16{"Pobierz", "Pobrano", "Czekaj"}."Czekaj", "error in (no error)"=w637) -> ("error out"=w636:errorcluster, "Flaga"=w638:bool, "Impulsy Out"=w635:dbl)  [unwired: 6 in, 1 out]
        }
        n260 = Bundle By Name(cluster=w624, "Wzorcowanie"=w622) -> (w623:T8)
        n261 = call "Enk_Skalowanie drogi GUI.vi"("error in (no error)"=w631, "Droga In"=w626) -> ("error out"=w630:errorcluster, "Skala"=w625:dbl)  [unwired: 8 in]
        "Skala" <- w625
        n262 = local write "Przemieszczenie"(w623) -> ()
        n263 = call "Skaluj wartosc enkodera FVG.vi"("Akcja (GET)"=FVG_akcje_podstawowa."SET", "error in (no error)"=w630, "Skala"=w625) -> ("error out"=w627:errorcluster)  [unwired: 7 in, 1 out]
      }
      event Value Change {
        n264 = event-data() -> ("NewVal"=w642:T8)  [unwired: 1 in, 5 out]
        n265 = Unbundle By Name(w642) -> ("Zerowanie"=w646:bool, "dT"=w645:dbl, "Kanał"=w644:T9)
        n266 = call "Przenies enkodery FVG.vi"("Akcja (Get)"=FVG_akcje_podstawowa."SET", "error in (no error)"=w648, "Kanał in"=w644, "dT in"=w645, "Zerowanie in"=w646) -> ("error out"=w647:errorcluster)  [unwired: 3 in, 3 out]
      }
      event Value Change {
        w664 = FVG_GUI_akcje."SET DI Aktywny" ("Akcja (Get)")
        n267 = event-data() -> ()  [unwired: 1 in, 6 out]
        n268 = Unbundle By Name("Kanały cyfrowe") -> ("DI1 Opis"=w659:string, "DI2 Opis"=w658:string, "DI3 Opis"=w657:string, "DI4 Opis"=w656:string)
        n269 = Build Array(w659, w658, w657, w656) -> (w652:string[])
        n270 = for {
          tunnel: w655 -> [w672] mode=indexing
          tunnel: [w671] -> w654
          tunnel: w653 -> [w670]
          tunnel: w652 -> [w669] mode=indexing
          n271 = property class="Bool (strict)"(reference=w672, error in=w670, "Caption.Text"=w669) -> (error out=w671:errorcluster)  [unwired: 1 out]
        }
        n272 = call "DI_parametry z kontrolki.vi"("Kanały cyfrowe in"="Kanały cyfrowe") -> ("Opisy out"=w661:string[], "Aktywne out"=w666:bool[], "Mnożniki out"=w665:dbl[])  [unwired: 7 in, 1 out]
        n273 = call "Przenies opisy FVG.vi"("Akcja (Get)"=w664, "error in (no error)"=w654, "DI opisy in"=w661) -> ("error out"=w662:errorcluster)  [unwired: 6 in, 2 out]
        n274 = call "Przenies aktywne FVG.vi"("Akcja (Get)"=w664, "error in (no error)"=w662, "DI Aktywne in"=w666) -> ("error out"=w667:errorcluster)  [unwired: 6 in, 2 out]
        n275 = call "Przenies mnozniki FVG.vi"("Akcja (Get)"=w664, "error in (no error)"=w667, "DI Mnozniki in"=w665) -> ("error out"=w663:errorcluster)  [unwired: 6 in, 2 out]
      }
      event Value Change {
        w674 = "Konfiguracja\\AI_konwersja.txt"  # name or relative path
        w679 = FALSE  # event data
        # "#todo dorobić automatyczne wyszukiwanie pliku"
        n276 = event-data() -> ()  [unwired: 1 in, 6 out]
        n277 = Index Array(array=w691, index=0) -> (element=w692:refnum<vi>)
        n278 = property class="Clust (strict)"(reference=w692, error in=w687) -> (reference out=w689:refnum<vi>, error out=w688:errorcluster, "Value"=w684:T13)
        n279 = Generate User Event(user event=w680, event data cluster=w679) -> ()  [unwired: 2 in, 2 out]
        n280 = call <vilib>:"Application Directory.vi"() -> ("Application Directory"=w675:path)
        n281 = Unbundle By Name(w684) -> ("Wartość"=w690:T14)
        n282 = Build Path(base path=w675, name or relative path=w674) -> (appended path=w673:path)
        n283 = call "Okno_Czytaj_konwersje.vi"("Path"=w673, "error in"=w688, "Wartosc In"=w690) -> ("error out"=w681:errorcluster, "Wartosc Out"=w685:T14)  [unwired: 7 in]
        n284 = Bundle By Name(cluster=w684, "Wartość"=w685) -> (w683:T13)
        n285 = property class="Clust (strict)"(reference=w689, error in=w681, "Value"=w683) -> (error out=w686:errorcluster)  [unwired: 1 out]
        n286 = call "Przenies mnozniki konw FVG.vi"("Akcja (GET)"=FVG_akwizycje_akcje."SET", "Przetwornik in"=w683) -> ()  [unwired: 8 in, 2 out]
      }
      event Value Change {
        w695 = "Konfiguracja\\AI_konwersja.txt"  # name or relative path
        w700 = FALSE  # event data
        # "#todo dorobić automatyczne wyszukiwanie pliku"
        n287 = event-data() -> ()  [unwired: 1 in, 6 out]
        n288 = Index Array(array=w712, index=2) -> (element=w713:refnum<vi>)
        n289 = property class="Clust (strict)"(reference=w713, error in=w708) -> (reference out=w710:refnum<vi>, error out=w709:errorcluster, "Value"=w705:T13)
        n290 = call <vilib>:"Application Directory.vi"() -> ("Application Directory"=w696:path)
        n291 = Generate User Event(user event=w701, event data cluster=w700) -> ()  [unwired: 2 in, 2 out]
        n292 = Unbundle By Name(w705) -> ("Wartość"=w711:T14)
        n293 = Build Path(base path=w696, name or relative path=w695) -> (appended path=w694:path)
        n294 = call "Okno_Czytaj_konwersje.vi"("Path"=w694, "error in"=w709, "Wartosc In"=w711) -> ("error out"=w702:errorcluster, "Wartosc Out"=w706:T14)  [unwired: 7 in]
        n295 = Bundle By Name(cluster=w705, "Wartość"=w706) -> (w704:T13)
        n296 = property class="Clust (strict)"(reference=w710, error in=w702, "Value"=w704) -> (error out=w707:errorcluster)  [unwired: 1 out]
        n297 = call "Przenies mnozniki konw FVG.vi"("Akcja (GET)"=FVG_akwizycje_akcje."SET", "Przetwornik in"=w704) -> ()  [unwired: 8 in, 2 out]
      }
      event Value Change {
        w716 = "Konfiguracja\\AI_konwersja.txt"  # name or relative path
        w721 = FALSE  # event data
        # "#todo dorobić automatyczne wyszukiwanie pliku"
        n298 = event-data() -> ()  [unwired: 1 in, 6 out]
        n299 = Index Array(array=w733, index=3) -> (element=w734:refnum<vi>)
        n300 = property class="Clust (strict)"(reference=w734, error in=w729) -> (reference out=w731:refnum<vi>, error out=w730:errorcluster, "Value"=w726:T13)
        n301 = call <vilib>:"Application Directory.vi"() -> ("Application Directory"=w717:path)
        n302 = Generate User Event(user event=w722, event data cluster=w721) -> ()  [unwired: 2 in, 2 out]
        n303 = Unbundle By Name(w726) -> ("Wartość"=w732:T14)
        n304 = Build Path(base path=w717, name or relative path=w716) -> (appended path=w715:path)
        n305 = call "Okno_Czytaj_konwersje.vi"("Path"=w715, "error in"=w730, "Wartosc In"=w732) -> ("error out"=w723:errorcluster, "Wartosc Out"=w727:T14)  [unwired: 7 in]
        n306 = Bundle By Name(cluster=w726, "Wartość"=w727) -> (w725:T13)
        n307 = property class="Clust (strict)"(reference=w731, error in=w723, "Value"=w725) -> (error out=w728:errorcluster)  [unwired: 1 out]
        n308 = call "Przenies mnozniki konw FVG.vi"("Akcja (GET)"=FVG_akwizycje_akcje."SET", "Przetwornik in"=w725) -> ()  [unwired: 8 in, 2 out]
      }
      event Value Change {
        w737 = "Konfiguracja\\AI_konwersja.txt"  # name or relative path
        w742 = FALSE  # event data
        # "#todo dorobić automatyczne wyszukiwanie pliku"
        n309 = event-data() -> ()  [unwired: 1 in, 6 out]
        n310 = Index Array(array=w754, index=4) -> (element=w755:refnum<vi>)
        n311 = property class="Clust (strict)"(reference=w755, error in=w750) -> (reference out=w752:refnum<vi>, error out=w751:errorcluster, "Value"=w747:T13)
        n312 = call <vilib>:"Application Directory.vi"() -> ("Application Directory"=w738:path)
        n313 = Generate User Event(user event=w743, event data cluster=w742) -> ()  [unwired: 2 in, 2 out]
        n314 = Unbundle By Name(w747) -> ("Wartość"=w753:T14)
        n315 = Build Path(base path=w738, name or relative path=w737) -> (appended path=w736:path)
        n316 = call "Okno_Czytaj_konwersje.vi"("Path"=w736, "error in"=w751, "Wartosc In"=w753) -> ("error out"=w744:errorcluster, "Wartosc Out"=w748:T14)  [unwired: 7 in]
        n317 = Bundle By Name(cluster=w747, "Wartość"=w748) -> (w746:T13)
        n318 = property class="Clust (strict)"(reference=w752, error in=w744, "Value"=w746) -> (error out=w749:errorcluster)  [unwired: 1 out]
        n319 = call "Przenies mnozniki konw FVG.vi"("Akcja (GET)"=FVG_akwizycje_akcje."SET", "Przetwornik in"=w746) -> ()  [unwired: 8 in, 2 out]
      }
      event Value Change {
        w758 = "Konfiguracja\\AI_konwersja.txt"  # name or relative path
        w763 = FALSE  # event data
        # "#todo dorobić automatyczne wyszukiwanie pliku"
        n320 = event-data() -> ()  [unwired: 1 in, 6 out]
        n321 = Index Array(array=w775, index=5) -> (element=w776:refnum<vi>)
        n322 = property class="Clust (strict)"(reference=w776, error in=w771) -> (reference out=w773:refnum<vi>, error out=w772:errorcluster, "Value"=w768:T13)
        n323 = call <vilib>:"Application Directory.vi"() -> ("Application Directory"=w759:path)
        n324 = Generate User Event(user event=w764, event data cluster=w763) -> ()  [unwired: 2 in, 2 out]
        n325 = Unbundle By Name(w768) -> ("Wartość"=w774:T14)
        n326 = Build Path(base path=w759, name or relative path=w758) -> (appended path=w757:path)
        n327 = call "Okno_Czytaj_konwersje.vi"("Path"=w757, "error in"=w772, "Wartosc In"=w774) -> ("error out"=w765:errorcluster, "Wartosc Out"=w769:T14)  [unwired: 7 in]
        n328 = Bundle By Name(cluster=w768, "Wartość"=w769) -> (w767:T13)
        n329 = property class="Clust (strict)"(reference=w773, error in=w765, "Value"=w767) -> (error out=w770:errorcluster)  [unwired: 1 out]
        n330 = call "Przenies mnozniki konw FVG.vi"("Akcja (GET)"=FVG_akwizycje_akcje."SET", "Przetwornik in"=w767) -> ()  [unwired: 8 in, 2 out]
      }
      event Value Change {
        w779 = "Konfiguracja\\AI_konwersja.txt"  # name or relative path
        w784 = FALSE  # event data
        # "#todo dorobić automatyczne wyszukiwanie pliku"
        n331 = event-data() -> ()  [unwired: 1 in, 6 out]
        n332 = Index Array(array=w796, index=6) -> (element=w797:refnum<vi>)
        n333 = property class="Clust (strict)"(reference=w797, error in=w792) -> (reference out=w794:refnum<vi>, error out=w793:errorcluster, "Value"=w789:T13)
        n334 = call <vilib>:"Application Directory.vi"() -> ("Application Directory"=w780:path)
        n335 = Generate User Event(user event=w785, event data cluster=w784) -> ()  [unwired: 2 in, 2 out]
        n336 = Unbundle By Name(w789) -> ("Wartość"=w795:T14)
        n337 = Build Path(base path=w780, name or relative path=w779) -> (appended path=w778:path)
        n338 = call "Okno_Czytaj_konwersje.vi"("Path"=w778, "error in"=w793, "Wartosc In"=w795) -> ("error out"=w786:errorcluster, "Wartosc Out"=w790:T14)  [unwired: 7 in]
        n339 = Bundle By Name(cluster=w789, "Wartość"=w790) -> (w788:T13)
        n340 = property class="Clust (strict)"(reference=w794, error in=w786, "Value"=w788) -> (error out=w791:errorcluster)  [unwired: 1 out]
        n341 = call "Przenies mnozniki konw FVG.vi"("Akcja (GET)"=FVG_akwizycje_akcje."SET", "Przetwornik in"=w788) -> ()  [unwired: 8 in, 2 out]
      }
      event Value Change {
        w800 = "Konfiguracja\\AI_konwersja.txt"  # name or relative path
        w805 = FALSE  # event data
        # "#todo dorobić automatyczne wyszukiwanie pliku"
        n342 = event-data() -> ()  [unwired: 1 in, 6 out]
        n343 = Index Array(array=w817, index=7) -> (element=w818:refnum<vi>)
        n344 = property class="Clust (strict)"(reference=w818, error in=w813) -> (reference out=w815:refnum<vi>, error out=w814:errorcluster, "Value"=w810:T13)
        n345 = Generate User Event(user event=w806, event data cluster=w805) -> ()  [unwired: 2 in, 2 out]
        n346 = call <vilib>:"Application Directory.vi"() -> ("Application Directory"=w801:path)
        n347 = Unbundle By Name(w810) -> ("Wartość"=w816:T14)
        n348 = Build Path(base path=w801, name or relative path=w800) -> (appended path=w799:path)
        n349 = call "Okno_Czytaj_konwersje.vi"("Path"=w799, "error in"=w814, "Wartosc In"=w816) -> ("error out"=w807:errorcluster, "Wartosc Out"=w811:T14)  [unwired: 7 in]
        n350 = Bundle By Name(cluster=w810, "Wartość"=w811) -> (w809:T13)
        n351 = property class="Clust (strict)"(reference=w815, error in=w807, "Value"=w809) -> (error out=w812:errorcluster)  [unwired: 1 out]
        n352 = call "Przenies mnozniki konw FVG.vi"("Akcja (GET)"=FVG_akwizycje_akcje."SET", "Przetwornik in"=w809) -> ()  [unwired: 8 in, 2 out]
      }
      event Value Change {
        w821 = "Konfiguracja\\AI_konwersja.txt"  # name or relative path
        w830 = FALSE  # event data
        # "#todo dorobić automatyczne wyszukiwanie pliku"
        n353 = event-data() -> ()  [unwired: 1 in, 6 out]
        n354 = Index Array(array=w826, index=1) -> (element=w839:refnum<vi>)
        n355 = property class="Clust (strict)"(reference=w839, error in=w828) -> (reference out=w837:refnum<vi>, error out=w836:errorcluster, "Value"=w834:T13)
        n356 = Generate User Event(user event=w827, event data cluster=w830) -> ()  [unwired: 2 in, 2 out]
        n357 = call <vilib>:"Application Directory.vi"() -> ("Application Directory"=w822:path)
        n358 = Unbundle By Name(w834) -> ("Wartość"=w838:T14)
        n359 = Build Path(base path=w822, name or relative path=w821) -> (appended path=w820:path)
        n360 = call "Okno_Czytaj_konwersje.vi"("Path"=w820, "error in"=w836, "Wartosc In"=w838) -> ("error out"=w831:errorcluster, "Wartosc Out"=w835:T14)  [unwired: 7 in]
        n361 = Bundle By Name(cluster=w834, "Wartość"=w835) -> (w833:T13)
        n362 = property class="Clust (strict)"(reference=w837, error in=w831, "Value"=w833) -> (error out=w829:errorcluster)  [unwired: 1 out]
        n363 = call "Przenies mnozniki konw FVG.vi"("Akcja (GET)"=FVG_akwizycje_akcje."SET", "Przetwornik in"=w833) -> ()  [unwired: 8 in, 2 out]
      }
      event "AI HW conf array in": Value Change {
        # "#todo tymczasowo - do usunięcia"
        n364 = event-data() -> ()  [unwired: 1 in, 6 out]
        n365 = Send Notification(notification="AI HW conf array in", notifier=w844, error in (no error)=w847) -> (notifier out=w843:refnum<notifier>, error out=w846:errorcluster)
      }
      event Value Change {
        # "T - załączono\nF - wyłączono"
        n366 = event-data() -> ("OldVal"=w857:bool, "NewVal"=w855:bool)  [unwired: 1 in, 4 out]
        n367 = Not(x=w857) -> (.not. x?=w856:bool)
        n368 = And(x=w856, y=w855) -> (x .and. y?=w854:bool)
        n369 = case shown="True" w855 {
          frame False {
          }
          frame True {
            n370 = local write "Tab Control"(T1."Rejestracja Szybka" ("Tab Control")) -> ()
          }
        }
        n371 = Unbundle By Name(w853) -> ("Śledzenie"=w850:enum16{"Obwiednia", "Migawka"}, "Czas"=w851:i32)
        n372 = call "Przenies param rej szybka FVG.vi"("Śledzenie In"=w850, "Czas In"=w851, "Start In"=w854, "Akcja"=FVG_akwizycje_akcje."SET") -> ()  [unwired: 3 in, 5 out]
      }
      event Value Change {
        # "T - załączono\nF - wyłączono"
        n373 = event-data() -> ("OldVal"=w876:bool, "NewVal"=w867:bool)  [unwired: 1 in, 4 out]
        n374 = Unbundle By Name(w866) -> ("Rej.1.Aktywny"=w875:bool, "Rej.2.Aktywny"=w874:bool, "Rej.3.Aktywny"=w873:bool, "Rej.4.Aktywny"=w872:bool, "Rej.5.Aktywny"=w871:bool, "Rej.6.Aktywny"=w870:bool, "Rej.7.Aktywny"=w869:bool, "Rej.8.Aktywny"=w868:bool)
        n375 = Not(x=w876) -> (.not. x?=w877:bool)
        n376 = Compound Arithmetic op=OR(w875, w874, w873, w872, w871, w870, w869, w868) -> (w863:bool)
        n377 = And(x=w877, y=w867) -> (x .and. y?=w865:bool)
        n378 = And(x=w863, y=w865) -> (x .and. y?=w864:bool)
        n379 = case shown="True" w863 {
          tunnel: w866 -> [w883 w886]
          tunnel: w865 -> [_ w885]
          frame False {
            n380 = Bundle By Name(cluster=w883, "WolnaStart"=FALSE) -> (w881:T3)
            n381 = property on="Rejestracja wolna" class="Clust (strict)"("Value"=w881) -> ()  [unwired: 2 in, 2 out]
            n382 = One Button Dialog(message="Nie wybrano kanałów\ndo rejestracji") -> ()  [unwired: 1 in, 1 out]
          }
          frame True {
            n383 = call "Przenies param rej wolna FVG.vi"("Wolna In"=w886, "Start In"=w885, "Akcja"=FVG_akwizycje_akcje."SET") -> ()  [unwired: 5 in, 4 out]
          }
        }
        n384 = case shown="False" w864 {
          frame False {
          }
          frame True {
            n385 = local write "Tab Control"(T1."Rejestracja Wolna" ("Tab Control")) -> ()
          }
        }
      }
      event "Tab Control": Value Change {
        n386 = event-data() -> ("NewVal"=w891:T1)  [unwired: 1 in, 5 out]
        n387 = Equal?(x=w891, y=T1."Program" ("Tab Control")) -> (x = y?=w890:bool)
        n388 = case shown="True" w890 {
          frame False {
          }
          frame True {
            n389 = Two Button Dialog(message="Ustawienia Programu,Tylko dla osób upoważnionych!") -> (T button?=w898:bool)  [unwired: 2 in]
            n390 = Select(t=T1."Program" ("Tab Control"), s=w898, f=T1."Konfiguracja" ("Tab Control")) -> (s? t:f=w895:T1)
            n391 = local write "Tab Control"(w895) -> ()
          }
        }
      }
      event "Szybka STOP": Value Change; User Event {
        n392 = event-data() -> ()  [unwired: 1 in, 3 out]
        n393 = local write "Tab Control"(T1."Konfiguracja" ("Tab Control")) -> ()
        n394 = Bundle By Name(cluster=w906, "SzybkaStart"=FALSE) -> (w902:T7)
        n395 = property on="Rejestracja szybka" class="Clust (strict)"(error in=w904, "Val(Sgnl)"=w902) -> (error out=w903:errorcluster)  [unwired: 1 in, 1 out]
      }
      event "Wolna STOP": Value Change {
        n396 = event-data() -> ()  [unwired: 1 in, 6 out]
        n397 = Bundle By Name(cluster=w915, "WolnaStart"=FALSE ("SzybkaStart")) -> (w912:T3)
        n398 = local write "Tab Control"(T1."Konfiguracja" ("Tab Control")) -> ()
        n399 = property on="Rejestracja wolna" class="Clust (strict)"(error in=w914, "Val(Sgnl)"=w912) -> (error out=w913:errorcluster)  [unwired: 1 in, 1 out]
      }
      event "ZapiszAI_DI": Value Change {
        n400 = event-data() -> ()  [unwired: 1 in, 6 out]
        n401 = call <vilib>:"Application Directory.vi"() -> ("Application Directory"=w921:path)
        n402 = Build Path(base path=w921, name or relative path="Konfiguracja\\AI_Konfiguracja.txt") -> (appended path=w928:path)
        n403 = call "Zapis_ustawien_AI.vi"("error in (no error)"=w926, "Referencje Array"=w924, "Plik konf in"=w928) -> ("error out"=w927:errorcluster)  [unwired: 7 in, 1 out]
        n404 = call "generuj_nazwe_pliku.vi"("Nazwa bazowa"="Konfiguracja\\DI_Konfiguracja.txt" ("name or relative path"), "Application Directory"=w921) -> ("appended path"=w919:path)  [unwired: 8 in, 1 out]
        n405 = call "Zapis_ustawien_DI.vi"("error in (no error)"=w927, "Kanały cyfrowe"=w923, "Plik konf in"=w919) -> ("error out"=w925:errorcluster)  [unwired: 7 in, 1 out]
      }
      event "WczytajAI_DI": Value Change {
        n406 = event-data() -> ()  [unwired: 1 in, 6 out]
        n407 = call <vilib>:"Application Directory.vi"() -> ("Application Directory"=w947:path)
        n408 = Build Path(base path=w947, name or relative path="Konfiguracja\\AI_Konfiguracja.txt") -> (appended path=w945:path)
        n409 = Build Path(base path=w947, name or relative path="Konfiguracja\\DI_Konfiguracja.txt") -> (appended path=w943:path)
        n410 = call "Wczytanie_ustawien_AI.vi"("error in (no error)"=w938, "AI referencje Array"=w941, "Plik konf in"=w945) -> ("error out"=w939:errorcluster, "AiParamsOut"=w937:T13[])  [unwired: 6 in, 1 out]
        n411 = for {
          tunnel: w940 -> [w954] mode=indexing
          tunnel: w939 -> [w953]
          tunnel: [w951] -> w944
          tunnel: w937 -> [w950] mode=indexing
          n412 = Unbundle By Name(w950) -> ("Aktywny"=w952:bool)
          n413 = property class="Bool (strict)"(reference=w954, error in=w953, "Value"=w952) -> (error out=w951:errorcluster)  [unwired: 1 out]
        }
        n414 = call "Wczytanie_ustawien_DI.vi"("error in (no error)"=w944, "Kanały cyfrowe in"=w942, "Plik konf in"=w943) -> ("error out"=w934:errorcluster)  [unwired: 7 in, 1 out]
        n415 = Generate User Event(user event=w936, event data cluster=TRUE ("event data"), error in=w934) -> (error out=w935:errorcluster)  [unwired: 1 in, 1 out]
      }
    }
    "Stan" <- w404
  }
  "Array" <- w12
  n416 = while {
    tunnel: w67 -> [w971]
    tunnel: [w969] -> _
    shift-right: [w966] -> _
    shift-left: T18 {"Analogowe"=[], "Cyfrowe"=[], "Zwarcie"=[], "Enkoder"=[{"t0"=timestamp(0 s since 1904-01-01), "dt"=0.0, "Y"=[]}, {"t0"=timestamp(0 s since 1904-01-01), "dt"=1.0, "Y"=[]}, {"t0"=timestamp(0 s since 1904-01-01), "dt"=0.0, "Y"=[]}]} ("Data out") -> [w965]
    shift-right: [w962] -> _
    shift-left: 0.0 -> [w963]
    tunnel: w62 -> [w964]
    tunnel: w52 -> [w961]
    shift-right: [w959] -> _
    shift-left: FALSE -> [w960]
    stop <- w968 stop-if-true
    # "Akwizycja Szybka"
    n417 = Dequeue Element(queue=w971, error in (no error)=w961) -> (queue out=w958:refnum<queue>, element=w967:T18, error out=w956:errorcluster)  [unwired: 1 in, 1 out]
    n418 = case shown="No Error" w956 {
      tunnel: w967 -> [w979 _]
      tunnel: [w977 w1014] -> w966
      tunnel: w965 -> [w980 w1014]
      tunnel: w956 -> [w992 _]
      tunnel: w963 -> [w990 w1013]
      tunnel: [w989 w1013] -> w962
      tunnel: w964 -> [w988 _]
      tunnel: w960 -> [w975 w1012]
      tunnel: [w973 w1012] -> w959
      frame No Error {
        w972 = 25000  # size(32000)
        # "#todo zmniejszono bufor do 20000 dla próbkowania 2kHz"
        n419 = call "Przenies param rej szybka FVG.vi"("error in (no error)"=w992, "Akcja"=FVG_akwizycje_akcje."GETr") -> ("error out"=w986:errorcluster, "Restart Out"=w976:bool, "Śledzenie Out"=w982:enum16{"Obwiednia", "Migawka"}, "Czas Out"=w981:i32)  [unwired: 5 in, 1 out]
        n420 = call "Szybka_puste tablice.vi"("Reset"=w976, "error in (no error)"=w986, "Bufor in"=w980, "Kanaly in"=w979) -> ("error out"=w985:errorcluster, "Kanaly out"=w987:T18)  [unwired: 6 in]
        n421 = case shown="True" "Szybka ZAKONCZ" {
          tunnel: w990 -> [_ w1007]
          tunnel: [0.0 w1004] -> w989
          tunnel: w981 -> [_ w1006]
          tunnel: w988 -> [_ w1002]
          frame False {
          }
          frame True {
            n422 = To Double Precision Float(number=w1006) -> (double precision float=w1005:dbl)
            n423 = Add(x=w1007, y=0.02) -> (x+y=w1004:dbl)
            n424 = Less Or Equal?(x=w1005, y=w1004) -> (x <= y?=w1003:bool)
            n425 = case shown="True" w1003 {
              tunnel: w1002 -> [_ w1010]
              frame False {
              }
              frame True {
                n426 = local write "Szybka ZAKONCZ"(FALSE ("Szybka ZAKONCZ")) -> ()
                n427 = Generate User Event(user event=w1010, event data cluster=TRUE ("event data")) -> ()  [unwired: 2 in, 2 out]
              }
            }
          }
        }
        "Slide" <- w989
        n428 = Select(t=w976, s=w976, f=w975) -> (s? t:f=w974:bool)
        n429 = call "Szybka_buforuj.vi"("size(32000)"=w972, "error in (no error)"=w985, "Bufor in"=w987, "Kanaly in"=w979) -> ("Bufor out"=w977:T18, "Enk rozm"=→"Enk rozm":i32)  [unwired: 5 in, 1 out]
        n430 = call "Szybka czas FVG.vi"("Zadany"=0.3) -> ("Elapsed?"=w984:bool)  [unwired: 9 in, 1 out]
        n431 = case shown="True" w984 {
          tunnel: w977 -> [_ w997]
          tunnel: w982 -> [_ w999]
          tunnel: w981 -> [_ w998]
          tunnel: w974 -> [w994 w995]
          tunnel: [w994 w996] -> w973
          frame False {
          }
          frame True {
            w996 = FALSE  # Restart Out
            # "wysyłaj do FVG GUI"
            n432 = call "Szybka na wysw FVG.vi"("Restart in"=w995, "Akcja (GET)"=FVG_akcje_podstawowa."SET" ("Akcja"), "Bufor in"=w997, "Czas in"=w998, "Śledzenie in"=w999) -> ()  [unwired: 2 in, 5 out]
          }
        }
      }
      frame Error {
        (unwired) waveform(dbl)[] []  # Kanaly Array
      }
    }
    n433 = Get Queue Status(queue=w958, error in (no error)=w956) -> (error out=w955:errorcluster, # elements in queue=→"# elements in szybka queue":i32)  [unwired: 1 in, 6 out]
    n434 = call "Stop FVG.vi"("error in (no error)"=w955) -> ("Stop out"=w970:bool, "error out"=w969:errorcluster)  [unwired: 9 in]
    n435 = Or(x=w969, y=w970) -> (x .or. y?=w968:bool)
  }
  n436 = while {
    tunnel: w66 -> [w1034]
    tunnel: [w1032] -> _
    shift-right: [w1029] -> _
    shift-left: w50 -> [w1028]
    shift-right: [w1027] -> _
    shift-left: w50 -> [w1026]
    shift-right: [w1025] -> _
    shift-left: cluster{"Kanały":i32[][], T5[]} {"Kanały"=[], []} ("Rej Param") -> [w1024]
    tunnel: w52 -> [w1023]
    shift-right: [w1019] -> _
    shift-left: w4 -> [w1018]
    stop <- w1031 stop-if-true
    # "Akwizycja Wolna"
    n437 = Dequeue Element(queue=w1034, error in (no error)=w1023) -> (queue out=w1021:refnum<queue>, element=w1030:T18, error out=w1016:errorcluster)  [unwired: 1 in, 1 out]
    n438 = case shown="No Error" w1016 {
      tunnel: w1030 -> [w1065 _]
      tunnel: w1016 -> [w1066 _]
      tunnel: [w1037 w1087] -> w1029
      tunnel: w1028 -> [w1043 w1087]
      tunnel: [w1038 w1086] -> w1027
      tunnel: w1026 -> [w1054 w1086]
      tunnel: [w1044 w1085] -> w1025
      tunnel: w1024 -> [w1052 w1085]
      frame No Error {
        w1035 = 2500.0  # sample rate (3200)
        w1036 = 25000  # size(32000)
        w1041 = T32 0 items=["Reset", "Sprawdz"] ("Czas Akcja (Sprawdz)")
        w1042 = T32 1 items=["Reset", "Sprawdz"] ("Czas Akcja (Sprawdz)")
        # "#todo zmniejszono sample rate do 2000 dla próbkowania 2kHz"
        # "#todo zmniejszono bufor do 25000 dla próbkowania 2,5kHz"
        n439 = call "Przenies param rej wolna FVG.vi"("error in (no error)"=w1066, "Akcja"=FVG_akwizycje_akcje."GETr") -> ("error out"=w1051:errorcluster, "Restart Out"=w1039:bool, "Wolna Out"=w1056:T3)  [unwired: 6 in, 1 out]
        n440 = Unbundle By Name(w1056) -> ("Okres"=w1048:dbl)
        n441 = call "Szybka_puste tablice.vi"("Reset"=w1039, "error in (no error)"=w1051, "Bufor in"=w1043, "Kanaly in"=w1065) -> ("error out"=w1050:errorcluster, "Kanaly out"=w1049:T18)  [unwired: 6 in]
        n442 = call "Wolna_generuj_analog_wektory.vi"("Przetworzone in"=w1054, "Wolna In"=w1056, "Restart In"=w1039) -> ("Przetworzone out"=w1055:T18, "Rej Param"=w1053:cluster{"Kanały":i32[][], T5[]})  [unwired: 6 in, 1 out]
        n443 = call "Szybka_buforuj.vi"("size(32000)"=w1036, "error in (no error)"=w1050, "Bufor in"=w1049, "Kanaly in"=w1065) -> ("error out"=w1063:errorcluster, "Bufor out"=w1064:T18)  [unwired: 5 in, 1 out]
        n444 = Select(t=w1053, s=w1039, f=w1052) -> (s? t:f=w1044:cluster{"Kanały":i32[][], T5[]})
        n445 = call "Wolna_sprawdz_buf_size.vi"("Okres in"=w1048, "error in (no error)"=w1063, "Data in"=w1064) -> ("error out"=w1062:errorcluster, "Data out"=w1061:T18, "bufor OK?"=w1059:bool, "Okres out"=w1060:dbl)  [unwired: 5 in]
        n446 = Select(t=w1041, s=w1039, f=w1042) -> (s? t:f=w1040:T32)
        n447 = call "Wolna_rozdziel_buf.vi"("sample rate (3200)"=w1035, "error in (no error)"=w1062, "Data in"=w1061, "bufor OK in"=w1059, "Okres in"=w1060) -> ("error out"=w1045:errorcluster, "Data out"=w1037:T18, "bufor OK out"=w1058:bool, "Wydzielone out"=w1057:T18)  [unwired: 3 in]
        n448 = case shown="True" w1058 {
          tunnel: [w1076 w1078] -> w1038
          tunnel: w1055 -> [w1076 w1084]
          tunnel: w1057 -> [_ w1083]
          tunnel: w1044 -> [_ w1082]
          tunnel: w1048 -> [_ w1081]
          tunnel: w1045 -> [_ w1080]
          frame False {
          }
          frame True {
            n449 = call "Wolna_przetwarzanie.vi"("Rej Param"=w1082, "Okres In"=w1081, "error in (no error)"=w1080, "Przetworzone in"=w1084, "Wydzielone in"=w1083) -> ("error out"=w1077:errorcluster, "Przetworzone out"=w1079:T18)  [unwired: 5 in]
            n450 = call "Wolna_ogranicz_ramke.vi"("error in (no error)"=w1077, "Bufor in"=w1079) -> ("Bufor out"=w1078:T18)  [unwired: 8 in, 1 out]
          }
        }
        n451 = disable-structure shown="Enabled" {
          disable-tunnel: w1037 -> [w1068 _]
          frame Disabled {
            # "#info podgląd powoduje zapychanie bufora"
            n452 = Unbundle By Name(w1068) -> ("Analogowe"=w1071:waveform(dbl)[], "Cyfrowe"=w1072:waveform(dbl)[], "Enkoder"=w1073:waveform(dbl)[])
            n453 = Build Array (concatenate)(w1071, w1072, w1073) -> (w1069:waveform(dbl)[])
            "Wolna buf" <- w1069
            n454 = Array Size(array=w1069) -> (size(s)=w1070:i32)
            n455 = property on="Wolna buf" class="WFGraph (strict)"("LegNumRows"=w1070) -> ()  [unwired: 2 in, 2 out]
          }
          frame Enabled {
          }
        }
        n456 = call "Wolna czas FVG.vi"("Czas Akcja (Sprawdz)"=w1040, "Zadany"=0.3) -> ("Elapsed?"=w1047:bool)  [unwired: 8 in, 1 out]
        n457 = case shown="True" w1047 {
          tunnel: w1038 -> [_ w1075]
          frame False {
          }
          frame True {
            n458 = call "Wolna na wysw FVG.vi"("Akcja (GET)"=FVG_akcje_podstawowa."SET" ("Akcja"), "Wolna in"=w1075) -> ()  [unwired: 8 in, 2 out]
          }
        }
      }
      frame Error {
      }
    }
    n459 = Get Queue Status(queue=w1021, error in (no error)=w1016) -> (error out=w1015:errorcluster, # elements in queue=→"# elements in  wolna queue":i32)  [unwired: 1 in, 6 out]
    n460 = Tick Count (ms)() -> (millisecond timer value=w1019:u32)
    n461 = call "Stop FVG.vi"("Stop if error (T)"=FALSE, "error in (no error)"=w1015) -> ("Stop out"=w1033:bool, "error out"=w1032:errorcluster)  [unwired: 8 in]
    n462 = Subtract(x=w1019, y=w1018) -> (x-y=→"wolna delay":u32)
    n463 = Or(x=w1032, y=w1033) -> (x .or. y?=w1031:bool)
  }
  n464 = while {
    shift-right: [w1130] -> _
    shift-left: _ -> [w1131]
    tunnel: w52 -> [w1124]
    shift-right: [w1100] -> _
    shift-left: w41 -> [w1103]
    stop <- w1126 stop-if-true
    (unwired) FALSE ("Stop in (F)")
    w1099 = FVG_akwizycje_akcje."GET" ("Akcja")
    # "#info liczy wartości\nskuteczną, średnią i\nwyprostowaną"
    # "0 - brak\n1 - szybka\n2 - wolna"
    # "Aktualizacja wykresow"
    n465 = Wait (ms)(milliseconds to wait=u32 400) -> ()  [unwired: 1 out]
    n466 = call "Przenies aktywne FVG.vi"() -> ("DI Aktywne out"=w1092:bool[], "AI Aktywne out"=w1113:bool[])  [unwired: 9 in, 1 out]
    n467 = call "Referencje Mem FVG.vi"() -> ("AI wskazniki array out"=w1107:refnum<vi>[], "DI wartosci array out"=w1094:refnum<vi>[], "AI aktywne array out"=w1108:refnum<vi>[], "AI_param array out"=w1101:refnum<vi>[])  [unwired: 8 in]
    n468 = call "Oblicz zakres SVG.vi"("napiecie progu Low (0,1V)"=0.2, "Akcja (SET)"=FVG_akcje_podstawowa."GET") -> ("Przetw out"=w1090:T18, "Przekroczone Low"=w1109:bool[], "Przekroczone High"=w1110:bool[])  [unwired: 6 in, 1 out]
    n469 = call "Przenies param rej wolna FVG.vi"("error in (no error)"=w1124, "Akcja"=w1099) -> ("error out"=w1122:errorcluster, "Start Out"=w1102:bool)  [unwired: 6 in, 2 out]
    n470 = call "Przenies param rej szybka FVG.vi"("Akcja"=w1099) -> ("Start Out"=w1100:bool)  [unwired: 6 in, 4 out]
    n471 = Unbundle By Name(w1090) -> ("Cyfrowe"=w1089:waveform(dbl)[])
    n472 = Build Array(w1100, w1102) -> (w1125:bool[])
    n473 = for {
      tunnel: w1113 -> [w1153] mode=indexing
      tunnel: w1108 -> [w1155] mode=indexing
      shift-right: [w1158] -> _
      shift-left: 0 -> [w1159]
      tunnel: w1110 -> [w1157]
      tunnel: w1109 -> [w1156]
      tunnel: w1107 -> [w1154] mode=indexing
      tunnel: [w1150] -> w1106 mode=indexing
      tunnel: w1090 -> [w1151]
      tunnel: w1101 -> [w1149] mode=indexing
      tunnel: "Pokaż wszystkie" -> [w1148]
      n474 = case shown="True" w1153 {
        tunnel: w1159 -> [w1161 w1170]
        tunnel: [w1161 w1177] -> w1158
        tunnel: w1157 -> [_ w1176]
        tunnel: w1156 -> [_ w1173]
        tunnel: w1155 -> [_ w1174]
        tunnel: w1151 -> [_ w1171]
        tunnel: [0.0 w1167] -> w1150
        tunnel: w1149 -> [_ w1165]
        frame False {
        }
        frame True {
          n475 = property class="Clust (strict)"(reference=w1165) -> ("Value"=w1166:T13)  [unwired: 1 in, 2 out]
          n476 = Index Array(array=w1176, index=w1170) -> (element=w1175:bool)
          n477 = Index Array(array=w1173, index=w1170) -> (element=w1172:bool)
          n478 = Unbundle By Name(w1171) -> ("Analogowe"=w1169:waveform(dbl)[])
          n479 = call "Koloruj wskazniki.vi"("High"=w1175, "Low"=w1172, "AI Refnum"=w1174) -> ()  [unwired: 8 in, 1 out]
          n480 = Unbundle By Name(w1166) -> ("Typ pomiaru"=w1164:T33)
          n481 = Index Array(array=w1169, index=w1170) -> (element=w1168:waveform(dbl))
          n482 = Increment(x=w1170) -> (x+1=w1177:i32)
          n483 = Type Cast(type=RejWol_typ."Wprost" ("Typ rejestracji"), x=w1164) -> (*(type *) &x=w1162:T5)
          n484 = call "Wolna_obliczenia.vi"("Wektor1 in"=w1168, "Typ rejestracji"=w1162) -> ("Value out"=w1167:dbl)  [unwired: 7 in, 2 out]
        }
      }
      n485 = Select(t=w1148, s=w1148, f=w1153) -> (s? t:f=w1152:bool)
      n486 = property class="DigNum (strict)"(reference=w1154, "Visible"=w1152) -> ()  [unwired: 1 in, 2 out]
    }
    n487 = Exclusive Or(1:w1100, 2:w1103) -> (0:w1104:bool)
    n488 = Boolean Array To Number(Boolean array=w1125) -> (number=w1123:u32)
    n489 = for {
      tunnel: w1094 -> [w1147] mode=indexing
      tunnel: "Pokaż wszystkie" -> [w1145]
      tunnel: w1092 -> [w1133] mode=indexing
      tunnel: [w1140] -> w1091 mode=indexing
      tunnel: w1089 -> [w1138]
      shift-right: [w1136] -> _
      shift-left: 0 -> [w1135]
      w1139 = 2.5  # prog
      # "#info próg dla wartości cyfrowych"
      n490 = Index Array(array=w1138, index=w1135) -> (element=w1137:waveform(dbl))
      n491 = Increment(x=w1135) -> (x+1=w1134:i32)
      n492 = Select(t=w1145, s=w1145, f=w1133) -> (s? t:f=w1146:bool)
      n493 = Unbundle By Name(w1137) -> ("Y"=w1142:dbl[])
      n494 = Select(t=w1134, s=w1133, f=w1135) -> (s? t:f=w1136:i32)
      n495 = property class="Bool (strict)"(reference=w1147, "Visible"=w1146) -> ()  [unwired: 1 in, 2 out]
      n496 = Array Size(array=w1142) -> (size(s)=w1144:i32)
      n497 = Decrement(x=w1144) -> (x-1=w1143:i32)
      n498 = Index Array(array=w1142, index=w1143) -> (element=w1141:dbl)
      n499 = Greater?(x=w1141, y=w1139) -> (0:w1140:bool)
    }
    n500 = case shown="2" w1123 {
      tunnel: w1104 -> [_ _ w1215]
      frame 0, Default {
      }
      frame 1 {
        # "SZYBKA"
        n501 = call "Szybka na wysw FVG.vi"() -> ("error out"=w1182:errorcluster, "Śledzenie out"=w1179:enum16{"Obwiednia", "Migawka"}, "Bufor out"=w1181:T18, "Czas Out"=w1180:i32, "Restart out"=w1183:bool)  [unwired: 7 in]
        n502 = call "Szybka na wysw FVG.vi"() -> ()  [unwired: 7 in, 5 out]
        n503 = case shown="\"Obwiednia\", Default" w1179 {
          tunnel: w1181 -> [w1200 w1208]
          tunnel: [w1198 w1208] -> w1189
          tunnel: [w1199 w1207] -> w1185
          tunnel: w1182 -> [w1197 w1207]
          frame "Obwiednia", Default {
            n504 = Unbundle By Name(w1200) -> ("Analogowe"=w1202:waveform(dbl)[])
            n505 = for {
              tunnel: w1202 -> [w1206] mode=indexing
              tunnel: [w1205] -> w1201 mode=indexing
              tunnel: [w1204] -> w1199
              tunnel: w1197 -> [w1203]
              n506 = call "Rej_szybka_obwiednia.vi"("error in (no error)"=w1203, "Wfm in"=w1206) -> ("error out"=w1204:errorcluster, "Wfm max out"=w1205:waveform(dbl))  [unwired: 7 in, 1 out]
            }
            n507 = Bundle By Name(cluster=w1200, "Analogowe"=w1201) -> (w1198:T18)
          }
          frame "Migawka" {
          }
        }
        n508 = To Double Precision Float(number=w1180) -> (double precision float=w1187:dbl)
        n509 = property on="Slide" class="Slide (strict)"("Scale.Maximum"=w1187, "Scale.Minimum"=0.0 ("Scale.Range:Minimum")) -> ()  [unwired: 2 in, 2 out]
        n510 = control-ref of="Szybka"() -> (w1188:refnum<vi>)
        n511 = case shown="True" w1183 {
          tunnel: w1189 -> [w1192 w1196]
          tunnel: w1185 -> [_ w1195]
          tunnel: [w1191 w1193] -> w1184
          frame False {
            n512 = call "kanaly to array.vi"("Kanaly"=w1192) -> ("Kanaly Array"=w1191:waveform(dbl)[])  [unwired: 9 in, 1 out]
          }
          frame True {
            n513 = control-ref of="Szybka"() -> (w1194:refnum<vi>)
            n514 = call "Mixed graph przypisanie osi.vi"("Wvm Ref in"=w1194, "error in (no error)"=w1195, "Data in"=w1196) -> ("Przebiegi Wfm"=w1193:waveform(dbl)[])  [unwired: 6 in, 2 out]
          }
        }
        "Szybka" <- w1184
        n515 = call "Wfm_rozmiar_do_skali.vi"("Bufor in"=w1189) -> ("Size (s)"=w1190:dbl)  [unwired: 10 in]
        n516 = call "Wfm_skaluj_osX.vi"("size(s)"=w1190, "Zakres wysw"="Zakres wysw szybka", "Waveform in"=w1188) -> ()  [unwired: 8 in, 1 out]
      }
      frame 2 {
        # "WOLNA"
        n517 = call "Wolna na wysw FVG.vi"() -> ("Wolna out"=w1214:T18)  [unwired: 10 in, 1 out]
        n518 = case shown="True" w1215 {
          tunnel: w1214 -> [w1217 w1220]
          tunnel: [w1216 w1219] -> w1209
          frame False {
            n519 = call "kanaly to array.vi"("Kanaly"=w1217) -> ("Kanaly Array"=w1216:waveform(dbl)[])  [unwired: 9 in, 1 out]
          }
          frame True {
            n520 = control-ref of="Wolna data"() -> (w1218:refnum<vi>)
            n521 = call "Mixed graph przypisanie osi.vi"("Wvm Ref in"=w1218, "Data in"=w1220) -> ("Przebiegi Wfm"=w1219:waveform(dbl)[])  [unwired: 7 in, 2 out]
          }
        }
        "Wolna data" <- w1209
        n522 = control-ref of="Wolna data"() -> (w1212:refnum<vi>)
        n523 = call "Wfm_rozmiar_do_skali.vi"("Bufor in"=w1214) -> ("Size (s)"=w1213:dbl)  [unwired: 10 in]
        n524 = call "Wfm_skaluj_osX.vi"("size(s)"=w1213, "Zakres wysw"="Zakres wysw wolna", "Waveform in"=w1212) -> ()  [unwired: 8 in, 1 out]
        n525 = Array Size(array=w1209) -> (size(s)=w1210:i32)
        n526 = property on="Wolna data" class="WFGraph (strict)"("LegNumRows"=w1210) -> ()  [unwired: 2 in, 2 out]
      }
    }
    n527 = Not(x=w1131) -> (.not. x?=w1130:bool)
    n528 = Index Array(array=w1091) -> (element #1=→"DI1":bool, element #2=→"DI2":bool, element #3=→"DI3":bool, element #4=→"DI4":bool)  [unwired: 4 in]
    n529 = call "Stop FVG.vi"("Stop in (F)"=FALSE, "error in (no error)"=w1122) -> ("Stop out"=w1128:bool, "error out"=w1127:errorcluster)  [unwired: 8 in]
    n530 = Index Array(array=w1106) -> (element #1=→"Kanał 1":dbl, element #2=→"Kanał 2":dbl, element #3=→"Kanał 3":dbl, element #4=→"Kanał 4":dbl, element #5=→"Kanał 5":dbl, element #6=→"Kanał 6":dbl, element #7=→"Kanał 7":dbl, element #8=→"Kanał 8":dbl)  [unwired: 8 in]
    n531 = Or(x=w1127, y=w1128) -> (x .or. y?=w1126:bool)
    "Boolean" <- w1131
  }
  n532 = call <vilib>:"Clear Errors.vi"("error in (no error)"=w88) -> ("error out"=w87:errorcluster)  [unwired: 5 in, 1 out]
  n533 = call "CONF digital clear.vi"("error in (no error)"=w87, "Digital ref out"=w95) -> ()  [unwired: 9 in, 1 out]
  n534 = call <vilib>:"Clear Errors.vi"("error in (no error)"=w79) -> ("error out"=w78:errorcluster)  [unwired: 5 in, 1 out]
  n535 = Release Notifier(notifier=w90, error in (no error)=w91) -> (error out=w14:errorcluster)  [unwired: 1 in, 2 out]
  n536 = call "ACQ stop and clear.vi"("error in (no error)"=w78, "Tasks ref in"=w80) -> ("error out"=w46:errorcluster)  [unwired: 9 in]
  n537 = call "Zapisz TDMS FVG.vi"("Akcja"=w13, "error in (no error)"=w14) -> ()  [unwired: 8 in, 2 out]
  n538 = call "Error monitor FVG.vi"("Akcja (SET)"=FVG_akcje_podstawowa."GET", "error in (no error)"=w46) -> ("error out"=w45:errorcluster, "Czasy Array"=→"Czasy Array":dbl[], "Error Array"=→"Error Array":errorcluster[])  [unwired: 7 in]
  n539 = Release Queue(queue=w70, error in (no error)=w45) -> (error out=w68:errorcluster)  [unwired: 1 in, 2 out]
  n540 = Release Queue(queue=w69, error in (no error)=w68) -> (error out=w2:errorcluster)  [unwired: 1 in, 2 out]
  n541 = case shown="True" FALSE {
    tunnel: w2 -> [_ w1221]
    frame False {
    }
    frame True {
      n542 = Quit LabVIEW(quit? (T)=w1221) -> ()
    }
  }
